vi "Station - Create New Station (SubVI).vi"(6 "Load?":bool, 8 "error constant":errorcluster, 10 "Test Type":u16(ring) items=["Please Select", "Triaxial Shear", "Triaxial UU", "Shearbox", "Permeability", "Consolidation (Stepped Loading)/Swelling", "Saturation (Incremental)", "User Defined", "UCT", "Isotropic Consolidation", "Swelling Pressure"], 11 "Station Name":string) -> (0 "error out":errorcluster, 2 "Station ID":string, 3 "ForceClose":bool=TRUE, 4 "Delete?":bool)   [LabVIEW 2019]
uses:
  Controls/Station name-state.ctl
  Controls/CreateStation - Data Structure.ctl
  Controls/Global - Device.vi
  Controls/Global - IP Address.vi
  Controls/Global - Data UDP.vi
  Controls/Global - Device Input.vi
  Controls/Global - Channel.vi
  Controls/Global - Unit.vi
panel:
  out "Device":string[](array[string])
  out "List":string[](array[string])
  in  "Cancel":bool
  in  "Delete":bool
  out "Sub Tab":T1(tab)
  in  "PP TS":u16(ring) caption="Vertical Load" items=["Please Select"]
  in  "Disp TS":u16(ring) caption="Back Pressure" items=["Please Select"]
  in  "LT TS":u16(ring) caption="Cell Pressure" items=["Please Select"]
  out "Unit PPT Triaxial Shear":string caption="Cell Pressure Transducer"
  out "Unit Disp Triaxial Shear":string caption="Cell Pressure Transducer"
  out "Unit LT Triaxial Shear":string caption="Cell Pressure Transducer"
  out "Unit VC Triaxial Shear":string caption="Cell Pressure Transducer"
  out "Unit BPT Triaxial Shear":string caption="Cell Pressure Transducer"
  out "Unit CPT Triaxial Shear":string caption="Cell Pressure Transducer"
  in  "VLC Triaxial Shear":u16(ring) caption="Vertical Load" items=["Please Select"]
  in  "BPC Triaxial Shear":u16(ring) caption="Back Pressure" items=["Please Select"]
  out "Disp Triaxial Shear":sgl caption="Displacement" format="%.3f"
  out "PPT Triaxial Shear":sgl caption="Pore Pressure"
  out "LT Triaxial Shear":sgl caption="Load"
  out "BPT Triaxial Shear":sgl caption="Back Pressure" format="%.3f"
  out "VC Triaxial Shear":sgl caption="Volume Change"
  out "CPT Triaxial Shear":sgl caption="Cell Pressure" format="%.3f"
  in  "VLC TS":u16(ring) caption="Vertical Load" items=["Please Select"]
  in  "BPC TS":u16(ring) caption="Back Pressure" items=["Please Select"]
  in  "CPC TS":u16(ring) caption="Cell Pressure" items=["Please Select"]
  in  "CPC Triaxial Shear":u16(ring) caption="Cell Pressure" items=["Please Select"]
  in  "PP TUU":u16(ring) caption="Vertical Load" items=["Please Select"]
  in  "Disp TUU":u16(ring) caption="Cell Pressure" items=["Please Select"]
  in  "VLC TUU":u16(ring) caption="Vertical Load" items=["Please Select"]
  in  "CPC TUU":u16(ring) caption="Cell Pressure" items=["Please Select"]
  out "Unit CPT Triaxial UU":string caption="Cell Pressure Transducer"
  out "Unit VLT Triaxial UU":string caption="Cell Pressure Transducer"
  out "Unit Disp Triaxial UU":string caption="Cell Pressure Transducer"
  out "Unit PPT Triaxial UU":string caption="Cell Pressure Transducer"
  in  "VLC Triaxial UU":u16(ring) caption="Vertical Load" items=["Please Select"]
  out "CPT Triaxial UU":sgl caption="Cell Pressure" format="%.5f"
  out "VLT Triaxial UU":sgl caption="Vertical Load" format="%.5f"
  out "PPT Triaxial UU":sgl caption="Pore Pressure" format="%.5f"
  out "Disp Triaxial UU":sgl caption="Displacement" format="%.5f"
  in  "CPC Triaxial UU":u16(ring) caption="Cell Pressure" items=["Please Select"]
  in  "HDisp Shearbox":u16(ring) caption="Horinzontal Load" items=["Please Select"]
  in  "HL Shearbox":u16(ring) caption="Vertical Load" items=["Please Select"]
  in  "VDisp Shearbox":u16(ring) caption="Horinzontal Load" items=["Please Select"]
  in  "VL Shearbox":u16(ring) caption="Vertical Load" items=["Please Select"]
  out "Unit LT Shearbox":string caption="Cell Pressure Transducer"
  out "Unit Disp Shearbox":string caption="Cell Pressure Transducer"
  out "Unit HLT Shearbox":string caption="Cell Pressure Transducer"
  out "Unit H Dis Shearbox":string caption="Cell Pressure Transducer"
  in  "HLC Shearbox":u16(ring) caption="Horinzontal Load" items=["Please Select"]
  out "LT Shearbox":sgl caption="V Load" format="%#.5f"
  out "Disp Shearbox":sgl caption="V Displacement" format="%#.5f"
  out "H Disp Shearbox":sgl caption="H Displacement" format="%#.5f"
  out "HLT Shearbox":sgl caption="H Load" format="%#.5f"
  in  "VLC Shearbox":u16(ring) caption="Vertical Load" items=["Please Select"]
  in  "OVC Permea":u16(ring) caption="Back Pressure 2" items=["Please Select"]
  in  "BP2 Permea":u16(ring) caption="Back Pressure" items=["Please Select"]
  in  "PP Permea":u16(ring) caption="Cell Pressure" items=["Please Select"]
  in  "IVC Permea":u16(ring) caption="Back Pressure 2" items=["Please Select"]
  in  "BP Permea":u16(ring) caption="Back Pressure" items=["Please Select"]
  in  "CP Permea":u16(ring) caption="Cell Pressure" items=["Please Select"]
  out "Unit CPT Permeability":string caption="Cell Pressure Transducer"
  out "Unit BPT Permeability":string caption="Cell Pressure Transducer"
  out "Unit IVC Permeability":string caption="Cell Pressure Transducer"
  out "Unit BPT2 Permeability":string caption="Cell Pressure Transducer"
  out "Unit OVC Permeability":string caption="Cell Pressure Transducer"
  out "Unit PPT Permeability":string caption="Cell Pressure Transducer"
  in  "BPC2 Permeability":u16(ring) caption="Drain Pressure" items=["Please Select"]
  in  "BPC Permeability":u16(ring) caption="Back Pressure" items=["Please Select"]
  out "BPT2 Permeability":sgl caption="Drain Pressure" format="%.5f"
  out "PPT Permeability":sgl caption="Pore Pressure" format="%.5f"
  out "OVC Permeability":sgl caption="Outlet VC" format="%.5f"
  out "BPT Permeability":sgl caption="Back Pressure" format="%.5f"
  out "IVC Permeability":sgl caption="Inlet VC" format="%.5f"
  out "CPT Permeability":sgl caption="Cell Pressure" format="%.5f"
  in  "CPC Permeability":u16(ring) caption="Cell Pressure" items=["Please Select"]
  in  "Disp Consol":u16(ring) caption="Vertical Load" items=["Please Select"]
  in  "LT Consol":u16(ring) caption="Vertical Load" items=["Please Select"]
  out "Unit LT Consolidation":string caption="Cell Pressure Transducer"
  out "Unit Disp Consolidation":string caption="Cell Pressure Transducer"
  out "Disp Consolidation":sgl caption="Displacement" format="%.5f"
  out "LT Consolidation":sgl caption="Load Tranducer" format="%.5f"
  in  "VLC Consolidation":u16(ring) caption="Vertical Load" items=["Please Select"]
  in  "VC Saturation":u16(ring) caption="Cell Pressure" items=["Please Select"]
  in  "PP Saturation":u16(ring) caption="Back Pressure" items=["Please Select"]
  in  "CP Saturation":u16(ring) caption="Cell Pressure" items=["Please Select"]
  in  "BP Saturation":u16(ring) caption="Back Pressure" items=["Please Select"]
  out "Unit CPT Saturation":string caption="Cell Pressure Transducer"
  out "Unit BPT Saturation":string caption="Cell Pressure Transducer"
  out "Unit VC Saturation":string caption="Cell Pressure Transducer"
  out "Unit PPT Saturation":string caption="Cell Pressure Transducer"
  out "CPT Saturation":sgl caption="Cell Pressure" format="%.1f"
  out "VC Saturation":sgl caption="Volume Change" format="%.1f"
  out "BPT Saturation":sgl caption="Back Pressure" format="%.1f"
  out "PPT Saturation":sgl caption="Pore pressure" format="%.1f"
  in  "CPC Saturation":u16(ring) caption="Cell Pressure" items=["Please Select"]
  in  "BPC Saturation":u16(ring) caption="Back Pressure" items=["Please Select"]
  in  "H Disp UD":u16(ring) caption="Horizontal Load" items=["Please Select"]
  in  "HL UD":u16(ring) caption="Vertical Load" items=["Please Select"]
  in  "VDisp UD":u16(ring) caption="Back Pressure 2" items=["Please Select"]
  in  "VL UD":u16(ring) caption="Back Pressure" items=["Please Select"]
  in  "VC2 UD":u16(ring) caption="Cell Pressure" items=["Please Select"]
  in  "BP2 UD":u16(ring) caption="Horizontal Load" items=["Please Select"]
  in  "PP UD":u16(ring) caption="Vertical Load" items=["Please Select"]
  in  "VC1 UD":u16(ring) caption="Back Pressure 2" items=["Please Select"]
  in  "BP UD":u16(ring) caption="Back Pressure" items=["Please Select"]
  in  "CP UD":u16(ring) caption="Cell Pressure" items=["Please Select"]
  out "HD User Defined":sgl caption="H Displacement" format="%.5f"
  out "HL User Defined":sgl caption="H Load" format="%.5f"
  out "VD User Defined":sgl caption="V Displacement" format="%.5f"
  out "VC2 User Defined":sgl caption="Volume Change 2" format="%.5f"
  out "VC1 User Defined":sgl caption="Volume Change 1" format="%.5f"
  out "VL User Defined":sgl caption="V Load" format="%.5f"
  out "BPT2 User Defined":sgl caption="Drain Pressure" format="%.5f"
  out "PWP User Defined":sgl caption="Pore Pressure" format="%.5f"
  out "BPT User Defined":sgl caption="Back Pressure" format="%.5f"
  out "CPT User Defined":sgl caption="Cell Pressure" format="%.5f"
  in  "HLC User Defined":u16(ring) caption="Horizontal Load" items=["Please Select"]
  in  "VLC User Defined":u16(ring) caption="Vertical Load" items=["Please Select"]
  in  "BPC2 User Defined":u16(ring) caption="Drain Pressure" items=["Please Select"]
  in  "BPC User Defined":u16(ring) caption="Back Pressure" items=["Please Select"]
  in  "CPC User Defined":u16(ring) caption="Cell Pressure" items=["Please Select"]
  out "Unit VL User Defined":string caption="Cell Pressure Transducer"
  out "Unit VD User Defined":string caption="Cell Pressure Transducer"
  out "Unit HL User Defined":string caption="Cell Pressure Transducer"
  out "Unit HD User Defined":string caption="Cell Pressure Transducer"
  out "Unit VC2 User Defined":string caption="Cell Pressure Transducer"
  out "Unit BPT2 User Defined":string caption="Cell Pressure Transducer"
  out "Unit PWP User Defined":string caption="Cell Pressure Transducer"
  out "Unit VC1 User Defined":string caption="Cell Pressure Transducer"
  out "Unit BPT User Defined":string caption="Cell Pressure Transducer"
  out "Unit CPT User Defined":string caption="Cell Pressure Transducer"
  in  "Disp UCT":u16(ring) caption="Vertical Load" items=["Please Select"]
  in  "LT UCT":u16(ring) caption="Vertical Load" items=["Please Select"]
  out "Unit LT UCT":string caption="Cell Pressure Transducer"
  out "Unit Disp UCT":string caption="Cell Pressure Transducer"
  out "Disp iUCT":sgl caption="Displacement"
  out "LT iUCT":sgl caption="Load Tranducer"
  in  "VLC UCT":u16(ring) caption="Vertical Load" items=["Please Select"]
  in  "VC IsoCons":u16(ring) caption="Cell Pressure" items=["Please Select"]
  in  "PP IsoCons":u16(ring) caption="Back Pressure" items=["Please Select"]
  in  "CP IsoCons":u16(ring) caption="Cell Pressure" items=["Please Select"]
  in  "BP IsoCons":u16(ring) caption="Back Pressure" items=["Please Select"]
  out "Unit CPT IsoCons":string caption="Cell Pressure Transducer"
  out "Unit BPT IsoCons":string caption="Cell Pressure Transducer"
  out "Unit VC IsoCons":string caption="Cell Pressure Transducer"
  out "Unit PPT IsoCons":string caption="Cell Pressure Transducer"
  out "CPT iIsoCons":sgl caption="Cell Pressure" format="%.1f"
  out "VC iIsoCons":sgl caption="Volume Change"
  out "BPT iIsoCons":sgl caption="Back Pressure"
  out "PPT iIsoCons":sgl caption="Pore pressure"
  in  "CPC IsoCons":u16(ring) caption="Cell Pressure" items=["Please Select"]
  in  "BPC IsoCons":u16(ring) caption="Back Pressure" items=["Please Select"]
  in  "VL SPres":u16(ring) caption="Cell Pressure" items=["Please Select"]
  in  "VS SPress":u16(ring) caption="Back Pressure" items=["Please Select"]
  out "Unit VL SP":string caption="Cell Pressure Transducer"
  out "Unit VS SP":string caption="Cell Pressure Transducer"
  out "VL SP":sgl caption="Vertical Load" format="%.1f"
  out "VS SP":sgl caption="Vertical Stress"
  in  "Save":bool
  # "Live Reading"
  # "Control"
  # "Display"
  # "Live Reading"
  # "Display"
  # "Control"
  # "Live Reading"
  # "Control"
  # "Display"
  # "Live Reading"
  # "Control"
  # "Display"
  # "Live Reading"
  # "Control"
  # "Display"
  # "Live Reading"
  # "Control"
  # "Display"
  # "Display"
  # "Control"
  # "Live Reading"
  # "Control"
  # "Display"
  # "Live Reading"
  # "Control"
  # "Display"
  # "Live Reading"
  # "Control"
  # "Display"
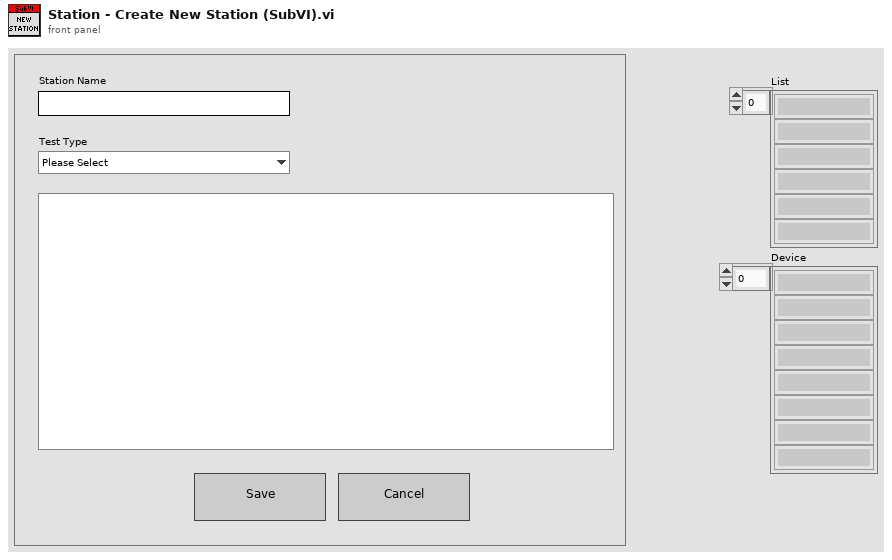
[diagram p1: front panel]
types:
  T1 = enum32{"Please Select", "Triaxial Shear", "Triaxial UU", "Shearbox", "Permeability", "Consolidation", "Saturation", "User Defined", "UCT", "Iso Consolidation", "Swelling Pressure"}
  T2 = enum16{"open", "replace", "create", "open or create", "replace or create", "replace or create with confirmation"}
  T3 = typedef "Station name-state.ctl" = enum16{"Init", "Idle", "Save", "Load", "Read", "Close"}
  T4 = typedef "CreateStation - Data Structure.ctl" = cluster{"Station Name":string[], "Station ID":i32}
  T5 = enum8{"Enabled", "Disabled", "Disabled and Grayed Out"}
  T6 = enum32{"Please Select", "Triaxial Shear", "Triaxial UU", "Shearbox", "Permeability", "Consolidation", "Saturation", "User Defined"}
  T7 = cluster{"Station Name":string, "Key Value":string[], "Key Names":string[]}[]
  T8 = typedef "UDP - Event.ctl" = u16
  T9 = typedef "UDP - Status.ctl" = u16
  T10 = cluster{"Channels":cluster{"Ch1":sgl, "Ch2":sgl, "Ch3":sgl, "Ch4":sgl, "Ch5":sgl, "Ch6":sgl, "Ch7":sgl, "Ch8":sgl, "Ch9":sgl, "Ch10":sgl, "Ch11":sgl, "Ch12":sgl, "Ch13":sgl, "Ch14":sgl, "Ch15":sgl, "Ch16":sgl}, "Event":T8, "Status":T9, "IP":string}[]
  T11 = cluster{"Name":string[], "Unit":string[], "Decimal Point":u8[], "Ch Log":u8[], "H Alarm":u8[], "L Alarm":u8[], "H Limit":sgl[], "L Limit":sgl[], "Filter":u8[], "Gain":u8[], "Calib Type":u32[]}[]
  T12 = cluster{"Channels":cluster{"Ch1":sgl, "Ch2":sgl, "Ch3":sgl, "Ch4":sgl, "Ch5":sgl, "Ch6":sgl, "Ch7":sgl, "Ch8":sgl, "Ch9":sgl, "Ch10":sgl, "Ch11":sgl, "Ch12":sgl, "Ch13":sgl, "Ch14":sgl, "Ch15":sgl, "Ch16":sgl}, "Event":T8, "Status":T9, "IP":string}
  T13 = cluster{"Name":string[], "Unit":string[], "Decimal Point":u8[], "Ch Log":u8[], "H Alarm":u8[], "L Alarm":u8[], "H Limit":sgl[], "L Limit":sgl[], "Filter":u8[], "Gain":u8[], "Calib Type":u32[]}
  T14 = cluster{"Ch1":sgl, "Ch2":sgl, "Ch3":sgl, "Ch4":sgl, "Ch5":sgl, "Ch6":sgl, "Ch7":sgl, "Ch8":sgl, "Ch9":sgl, "Ch10":sgl, "Ch11":sgl, "Ch12":sgl, "Ch13":sgl, "Ch14":sgl, "Ch15":sgl, "Ch16":sgl}
  T15 = cluster{"Station Name":string, "Key Value":string[], "Key Names":string[]}
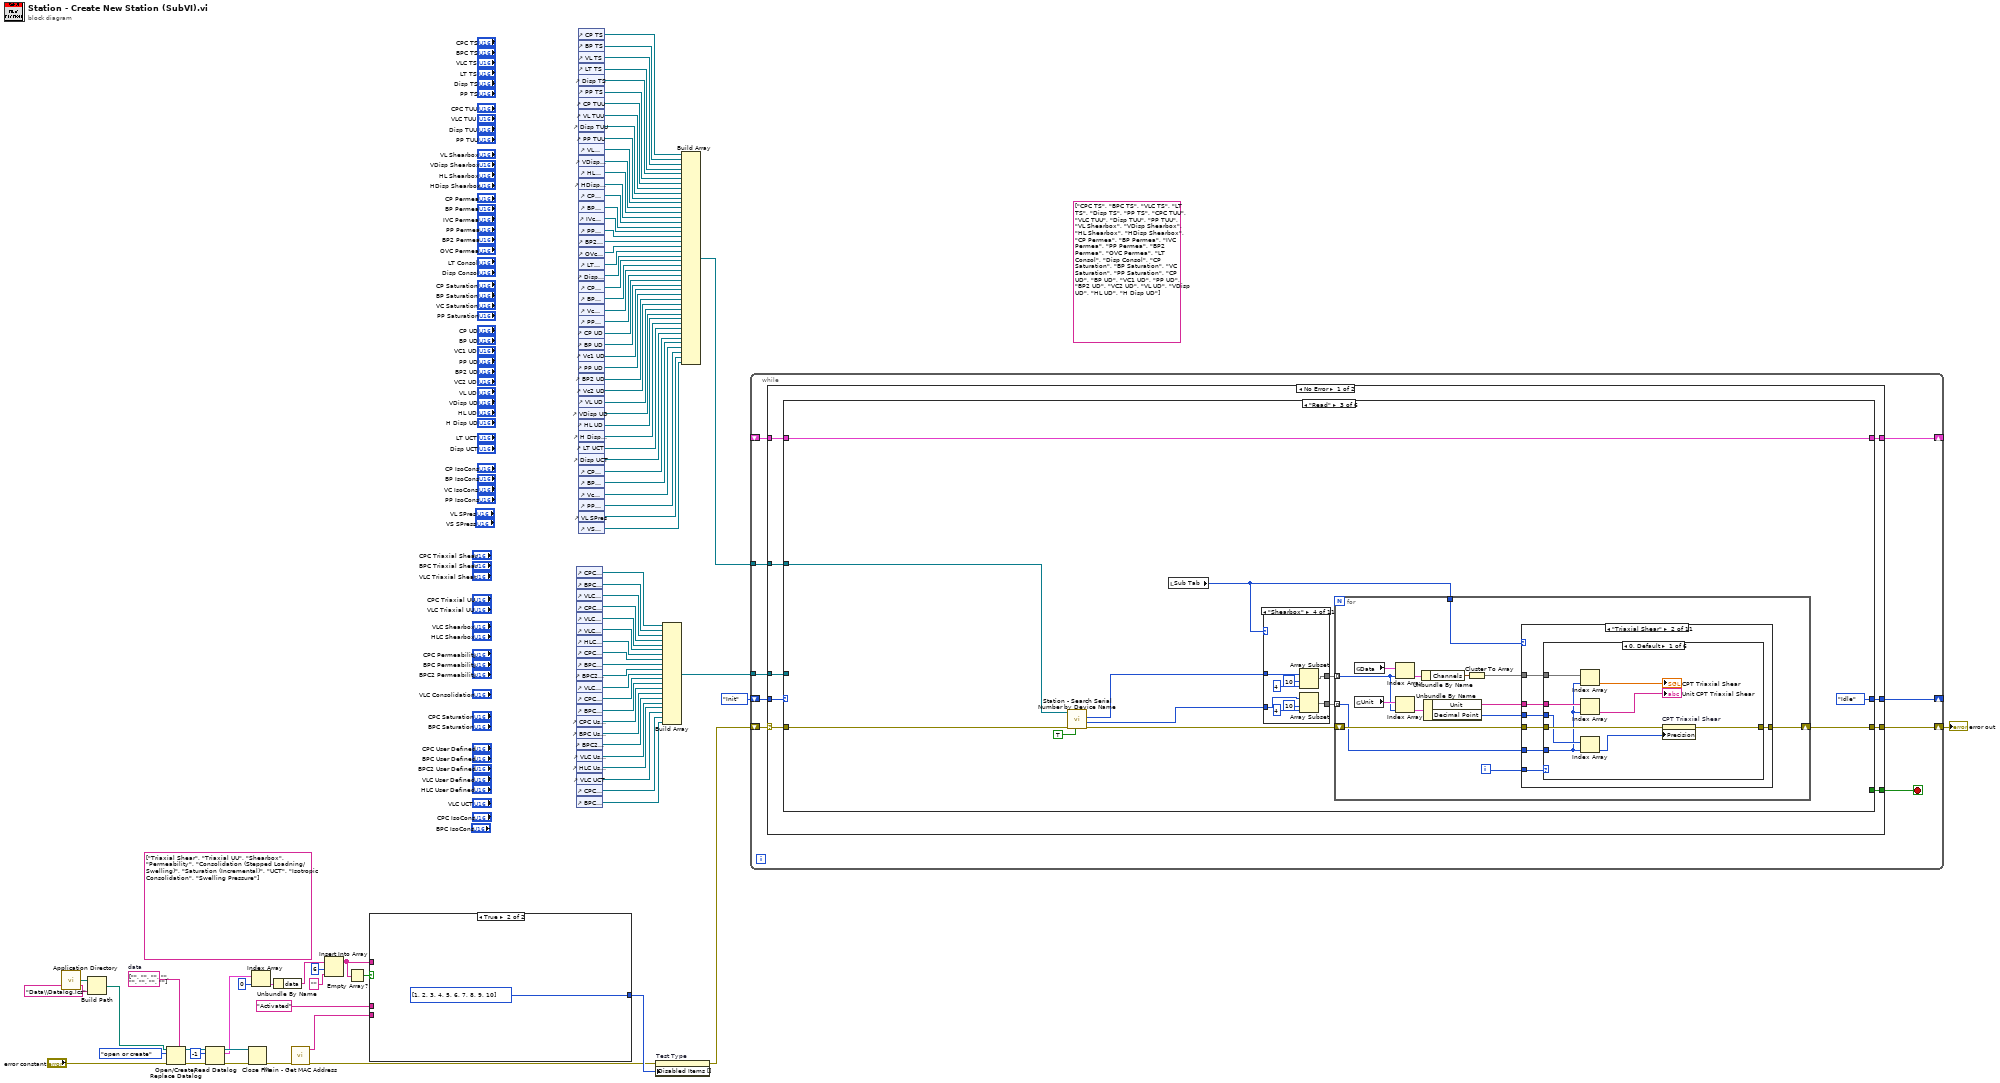
[diagram p0: block diagram]
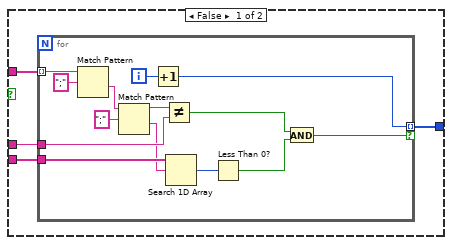
[diagram p2: hidden frame]
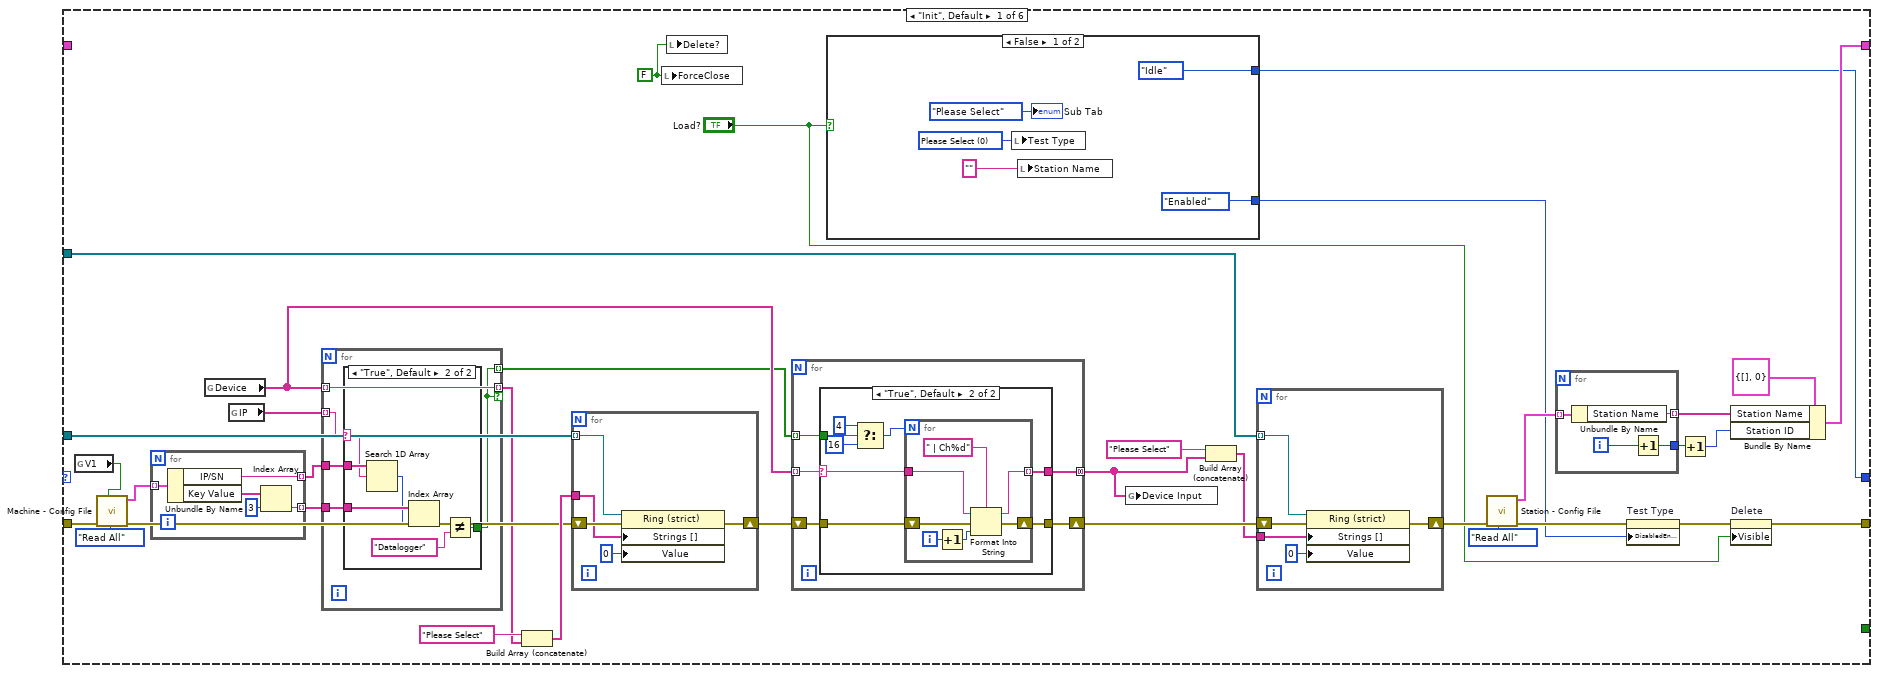
[diagram p3: hidden frame]
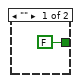
[diagram p4: hidden frame]
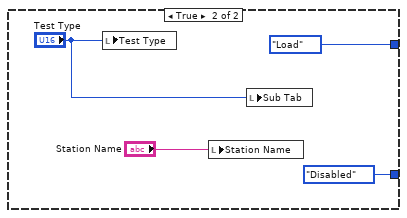
[diagram p5: hidden frame]
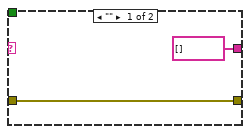
[diagram p6: hidden frame]
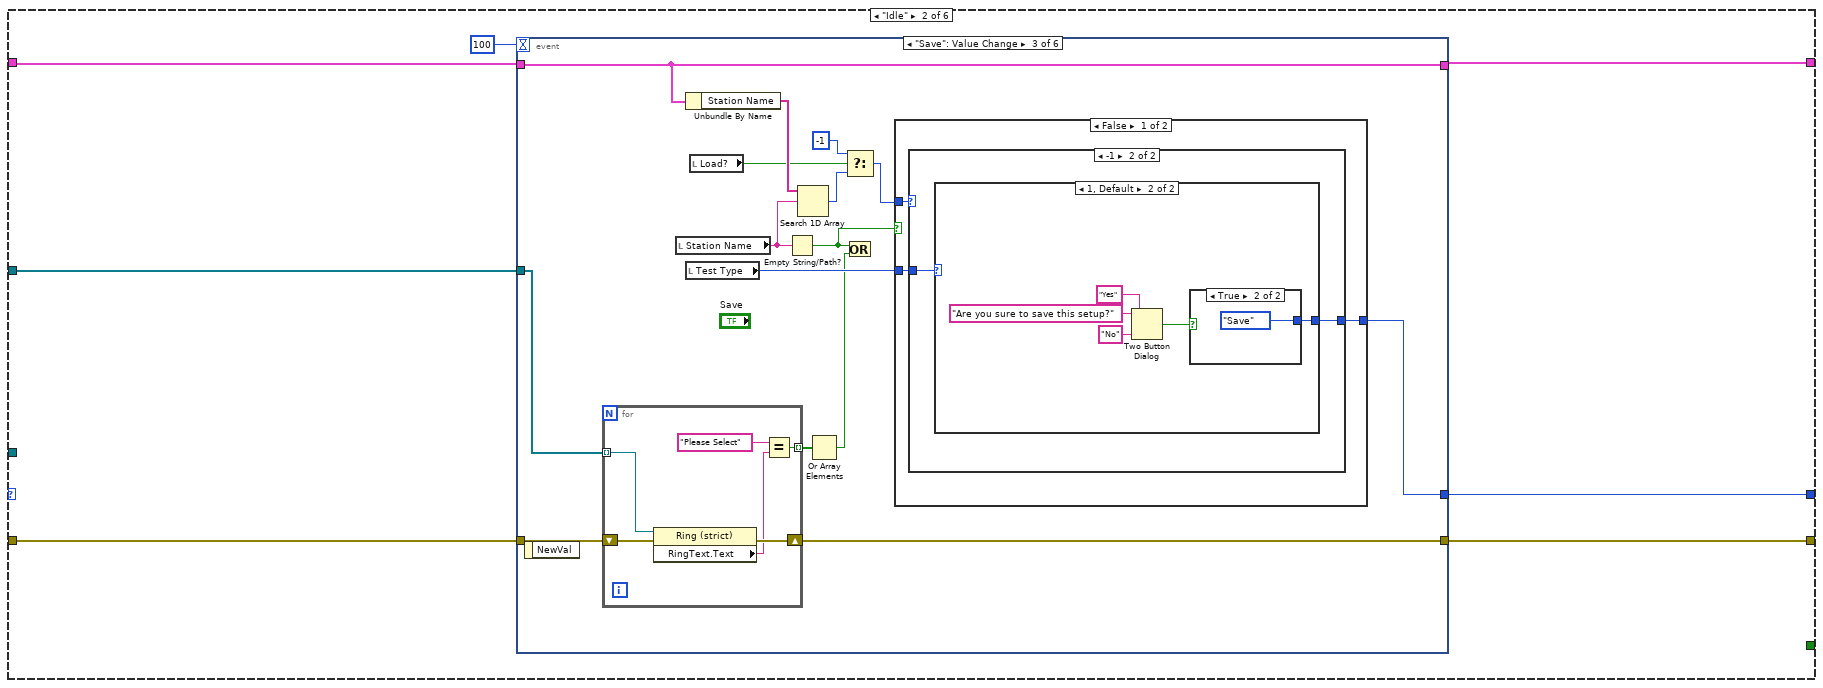
[diagram p7: hidden frame]
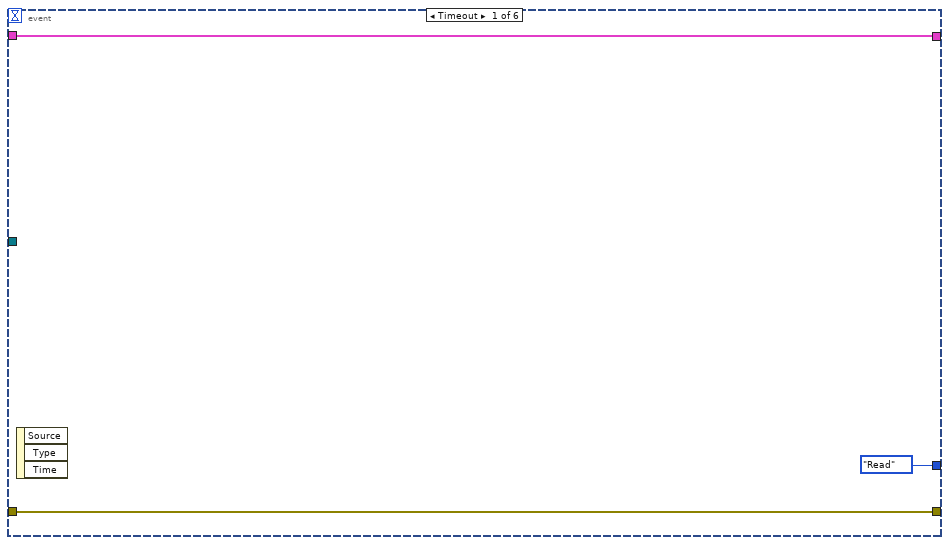
[diagram p8: hidden frame]
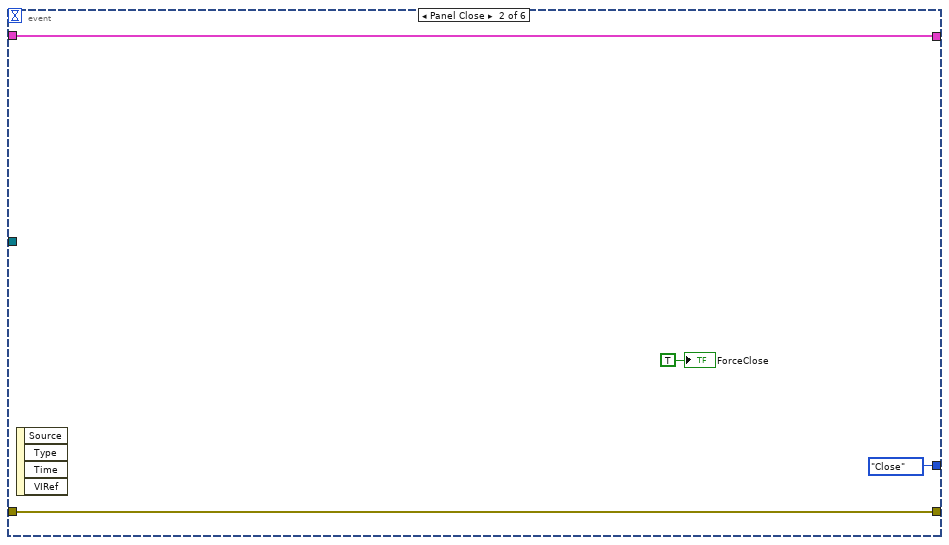
[diagram p9: hidden frame]
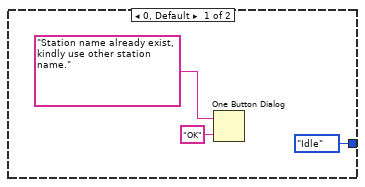
[diagram p10: hidden frame]
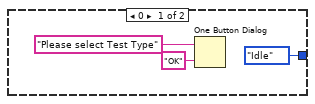
[diagram p11: hidden frame]
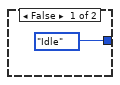
[diagram p12: hidden frame]
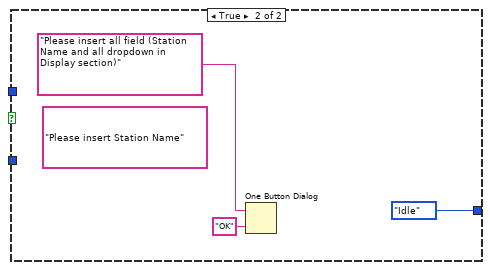
[diagram p13: hidden frame]
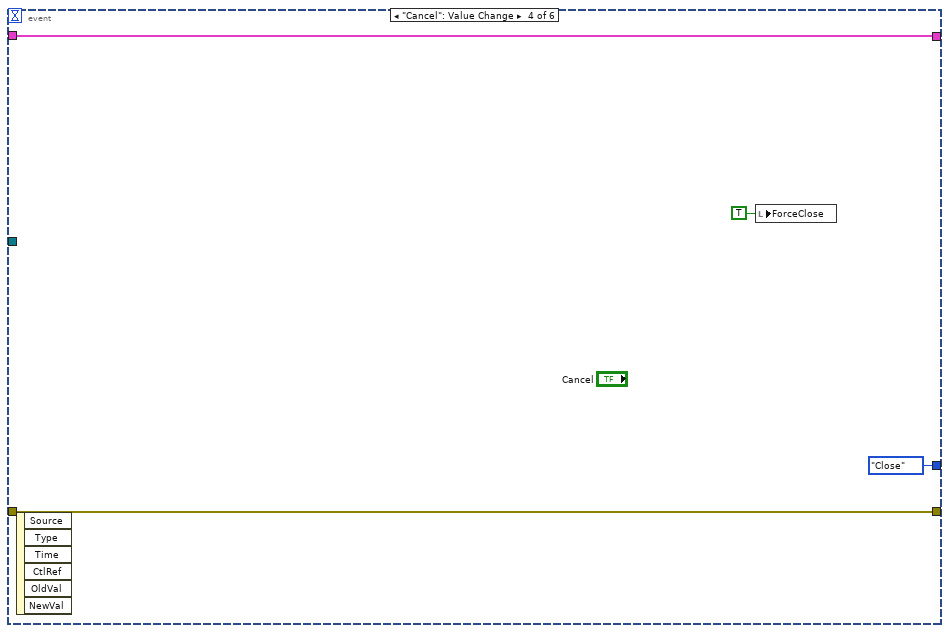
[diagram p14: hidden frame]
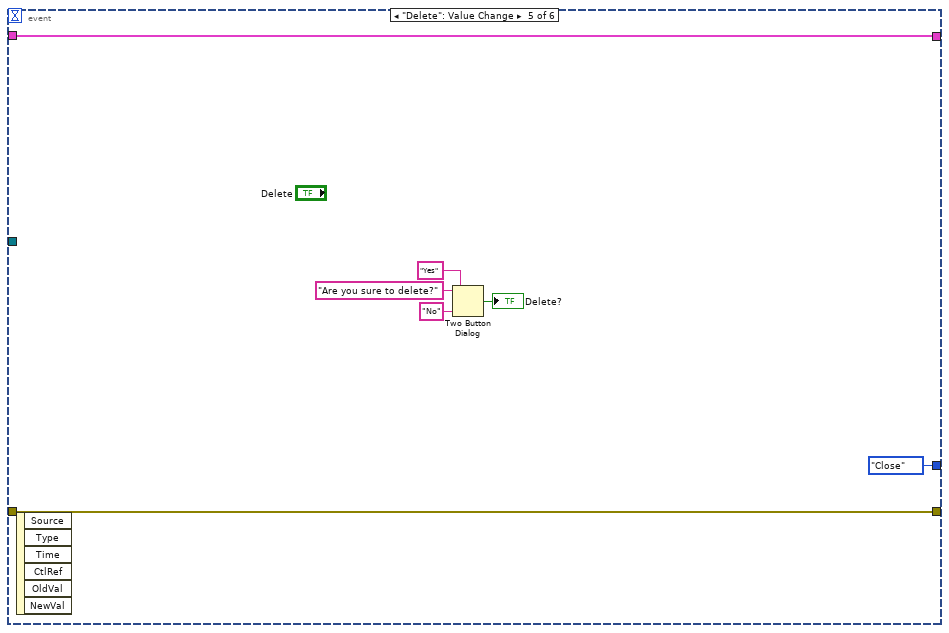
[diagram p15: hidden frame]
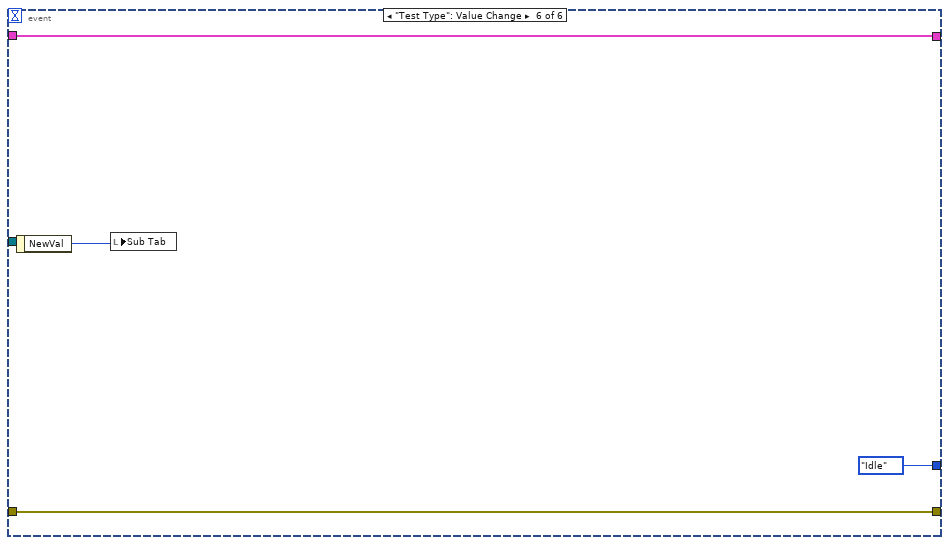
[diagram p16: hidden frame]
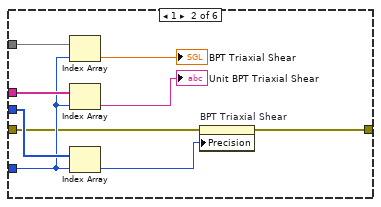
[diagram p18: hidden frame]
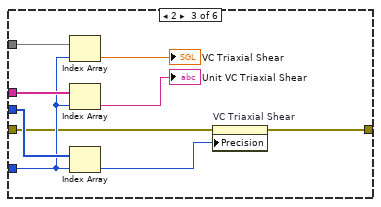
[diagram p19: hidden frame]
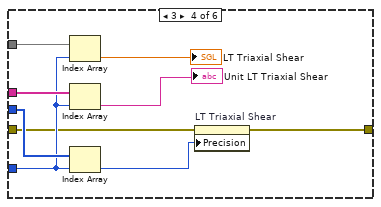
[diagram p20: hidden frame]
diagram:
  (unwired) string[] ["Triaxial Shear", "Triaxial UU", "Shearbox", "Permeability", "Consolidation (Stepped Loadning/Swelling)", "Saturation (Incremental)", "UCT", "Isotropic Consolidation", "Swelling Pressure"]
  w23 = string[] ["", "", "", "", "", "", "", ""]  # data
  (unwired) string[] ["CPC TS", "BPC TS", "VLC TS", "LT TS", "Disp TS", "PP TS", "CPC TUU", "VLC TUU", "Disp TUU", "PP TUU", "VL Shearbox", "VDisp Shearbox", "HL Shearbox", "HDisp Shearbox", "CP Permea", "BP Permea", "IVC Permea", "PP Permea", "BP2 Permea", "OVC Permea", "LT Consol", "Disp Consol", "CP Saturation", "BP Saturation", "VC Saturation", "PP Saturation", "CP UD", "BP UD", "VC1 UD", "PP UD", "BP2 UD", "VC2 UD", "VL UD", "VDisp UD", "HL UD", "H Disp UD"] ("Array")
  n1 = call <vilib>:"Application Directory.vi"() -> ("Application Directory"=w27:path)
  n2 = Build Path(base path=w27, name or relative path="Data\\Datalog.lcs") -> (appended path=w15:path)
  n3 = Open/Create/Replace Datalog(5:w23, 8:"error constant", 10:T2."open or create" ("operation (0:open)"), 11:w15) -> (0:w25:errorcluster, 3:w22:refnum<k1>)  [unwired: 2 in, 1 out]
  n4 = Read Datalog(4:w25, 6:-1 ("count (1)"), 7:w22) -> (0:w24:errorcluster, 2:w18:cluster{"data":string[]}[], 3:w21:refnum<k1>)
  n5 = Close File(refnum=w21, error in=w24) -> (error out=w5:errorcluster)  [unwired: 1 out]
  n6 = Index Array(array=w18, index=0) -> (element=w16:cluster{"data":string[]})
  n7 = Unbundle By Name(w16) -> ("data"=w10:string[])
  n8 = call "Main - Get MAC Address.vi"("error in (no error)"=w5) -> ("error out"=w4:errorcluster, "MAC Address"=w3:string[])  [unwired: 9 in]
  n9 = Insert Into Array(array=w10, index=6, new element="" ("new element/subarray")) -> (w7:string[])
  n10 = Empty Array?(array=w7) -> (empty?=w6:bool)
  n11 = case shown="True" w6 {
    tunnel: "Activated" -> [w98 _]
    tunnel: [w97 i32[] [1, 2, 3, 4, 5, 6, 7, 8, 9, 10]] -> w11
    tunnel: w7 -> [w96 _]
    tunnel: w3 -> [w95 _]
    frame False {
      n12 = for {
        tunnel: w96 -> [w108] mode=indexing
        tunnel: w98 -> [w112]
        tunnel: [w110] -> w97 mode=indexing if=w99
        tunnel: w95 -> [w104]
        i -> [w111]
        n13 = Match Pattern(string=w108, regular expression=";") -> (after substring=w106:string)  [unwired: 1 in, 3 out]
        n14 = Match Pattern(string=w106, regular expression=";") -> (before substring=w105:string, after substring=w103:string)  [unwired: 1 in, 2 out]
        n15 = Increment(x=w111) -> (x+1=w110:i32)
        n16 = Not Equal?(x=w105, y=w112) -> (x != y?=w100:bool)
        n17 = Search 1D Array(1D array=w104, element=w103) -> (index of element=w102:i32)  [unwired: 1 in]
        n18 = Less Than 0?(x=w102) -> (x < 0?=w101:bool)
        n19 = And(x=w100, y=w101) -> (x .and. y?=w99:bool)
      }
    }
    frame True {
    }
  }
  n20 = control-ref of="CPC Triaxial Shear"() -> (w93:refnum<vi>)
  n21 = control-ref of="BPC Triaxial Shear"() -> (w92:refnum<vi>)
  n22 = control-ref of="VLC Triaxial Shear"() -> (w91:refnum<vi>)
  n23 = control-ref of="CPC Triaxial UU"() -> (w90:refnum<vi>)
  n24 = control-ref of="VLC Triaxial UU"() -> (w89:refnum<vi>)
  n25 = control-ref of="VLC Shearbox"() -> (w88:refnum<vi>)
  n26 = control-ref of="HLC Shearbox"() -> (w87:refnum<vi>)
  n27 = control-ref of="CPC Permeability"() -> (w86:refnum<vi>)
  n28 = control-ref of="BPC Permeability"() -> (w85:refnum<vi>)
  n29 = control-ref of="BPC2 Permeability"() -> (w84:refnum<vi>)
  n30 = control-ref of="VLC Consolidation"() -> (w83:refnum<vi>)
  n31 = control-ref of="CPC Saturation"() -> (w82:refnum<vi>)
  n32 = control-ref of="BPC Saturation"() -> (w81:refnum<vi>)
  n33 = control-ref of="CPC User Defined"() -> (w80:refnum<vi>)
  n34 = control-ref of="BPC User Defined"() -> (w79:refnum<vi>)
  n35 = control-ref of="BPC2 User Defined"() -> (w78:refnum<vi>)
  n36 = control-ref of="VLC User Defined"() -> (w77:refnum<vi>)
  n37 = control-ref of="HLC User Defined"() -> (w76:refnum<vi>)
  n38 = control-ref of="VLC UCT"() -> (w36:refnum<vi>)
  n39 = control-ref of="CPC IsoCons"() -> (w35:refnum<vi>)
  n40 = control-ref of="BPC IsoCons"() -> (w34:refnum<vi>)
  n41 = control-ref of="CP TS"() -> (w75:refnum<vi>)
  n42 = control-ref of="BP TS"() -> (w74:refnum<vi>)
  n43 = control-ref of="VL TS"() -> (w73:refnum<vi>)
  n44 = control-ref of="LT TS"() -> (w72:refnum<vi>)
  n45 = control-ref of="Disp TS"() -> (w71:refnum<vi>)
  n46 = control-ref of="PP TS"() -> (w70:refnum<vi>)
  n47 = control-ref of="CP TUU"() -> (w69:refnum<vi>)
  n48 = control-ref of="VL TUU"() -> (w68:refnum<vi>)
  n49 = control-ref of="Disp TUU"() -> (w67:refnum<vi>)
  n50 = control-ref of="PP TUU"() -> (w66:refnum<vi>)
  n51 = control-ref of="VL Shearbox"() -> (w65:refnum<vi>)
  n52 = control-ref of="VDisp Shearbox"() -> (w64:refnum<vi>)
  n53 = control-ref of="HL Shearbox"() -> (w63:refnum<vi>)
  n54 = control-ref of="HDisp Shearbox"() -> (w62:refnum<vi>)
  n55 = control-ref of="CP Permea"() -> (w61:refnum<vi>)
  n56 = control-ref of="BP Permea"() -> (w60:refnum<vi>)
  n57 = control-ref of="IVc Permea"() -> (w59:refnum<vi>)
  n58 = control-ref of="PP Permea"() -> (w58:refnum<vi>)
  n59 = control-ref of="BP2 Permea"() -> (w57:refnum<vi>)
  n60 = control-ref of="OVc Permea"() -> (w56:refnum<vi>)
  n61 = control-ref of="LT Consol"() -> (w55:refnum<vi>)
  n62 = control-ref of="Disp Consol"() -> (w54:refnum<vi>)
  n63 = control-ref of="CP Saturation"() -> (w53:refnum<vi>)
  n64 = control-ref of="BP Saturation"() -> (w52:refnum<vi>)
  n65 = control-ref of="Vc Saturation"() -> (w51:refnum<vi>)
  n66 = control-ref of="PP Saturation"() -> (w50:refnum<vi>)
  n67 = control-ref of="CP UD"() -> (w49:refnum<vi>)
  n68 = control-ref of="BP UD"() -> (w48:refnum<vi>)
  n69 = control-ref of="Vc1 UD"() -> (w47:refnum<vi>)
  n70 = control-ref of="PP UD"() -> (w46:refnum<vi>)
  n71 = control-ref of="BP2 UD"() -> (w45:refnum<vi>)
  n72 = control-ref of="Vc2 UD"() -> (w44:refnum<vi>)
  n73 = control-ref of="VL UD"() -> (w43:refnum<vi>)
  n74 = control-ref of="VDisp UD"() -> (w42:refnum<vi>)
  n75 = control-ref of="HL UD"() -> (w41:refnum<vi>)
  n76 = control-ref of="H Disp UD"() -> (w40:refnum<vi>)
  n77 = control-ref of="LT UCT"() -> (w33:refnum<vi>)
  n78 = control-ref of="Disp UCT"() -> (w32:refnum<vi>)
  n79 = control-ref of="CP IsoCons"() -> (w31:refnum<vi>)
  n80 = control-ref of="BP IsoCons"() -> (w30:refnum<vi>)
  n81 = control-ref of="Vc IsoCons"() -> (w29:refnum<vi>)
  n82 = control-ref of="PP IsoCons"() -> (w28:refnum<vi>)
  n83 = control-ref of="VL SPres"() -> (w2:refnum<vi>)
  n84 = control-ref of="VS SPress"() -> (w1:refnum<vi>)
  n85 = property on="Test Type" class="Ring (strict)"(error in=w4, "Disabled Items []"=w11) -> (error out=w13:errorcluster)  [unwired: 1 in, 1 out]
  n86 = Build Array(w93, w92, w91, w90, w89, w88, w87, w86, w85, w84, w83, w82, w81, w80, w79, w78, w77, w76, w36, w35, w34) -> (w94:refnum<vi>[])
  n87 = Build Array(w75, w74, w73, w72, w71, w70, w69, w68, w67, w66, w65, w64, w63, w62, w61, w60, w59, w58, w57, w56, w55, w54, w53, w52, w51, w50, w49, w48, w47, w46, w45, w44, w43, w42, w41, w40, w33, w32, w31, w30, w29, w28, w2, w1) -> (w39:refnum<vi>[])
  n88 = while {
    shift-right: [w121] -> w37
    shift-left: w13 -> [w122]
    shift-right: [w119] -> _
    shift-left: Station_name-state."Init" -> [w120]
    shift-right: [w118] -> _
    shift-left: _ -> [w117]
    tunnel: w94 -> [w115]
    tunnel: w39 -> [w114]
    stop <- w116 stop-if-true
    n89 = case shown="No Error" w122 {
      selector: w122 -> [w131 w1207]
      tunnel: [w130 w1207] -> w121
      tunnel: w120 -> [w129 _]
      tunnel: [w128 _] -> w119
      tunnel: [w127 _] -> w118
      tunnel: w117 -> [w126 _]
      tunnel: [w125 _] -> w116
      tunnel: w115 -> [w124 _]
      tunnel: w114 -> [w123 _]
      frame No Error {
        n90 = case shown="\"Read\"" w129 {
          tunnel: w131 -> [w139 w236 w310 w896 w1055 w1206]
          tunnel: [w146 w235 w307 w902 w1052 w1206] -> w130
          tunnel: [w150 w234 Station_name-state."Idle" w901 Station_name-state."Idle" Station_name-state."Close"] -> w128
          tunnel: [w162 w232 w312 w886 w1053 T4 {"Station Name"=[], "Station ID"=0}] -> w127
          tunnel: w126 -> [_ w233 w312 w886 w1053 _]
          tunnel: [_ _ _ _ _ TRUE] -> w125
          tunnel: w124 -> [w166 _ _ w895 w1050 _]
          tunnel: w123 -> [w155 w230 w304 w877 w1049 _]
          frame "Init", Default {
            w144 = FALSE ("ForceClose")
            n91 = global read "Global - Data UDP.vi" "V1"() -> (w132:bool)
            n92 = call "Machine - Config File.vi"("Action"=enum16{"Write", "Read", "Read All", "Remove"}."Read All", "V1"=w132, "error in (no error)"=w139) -> ("error out"=w140:errorcluster, "Value Out"=w142:cluster{"IP/SN":string, "Key Value":string[]}[])  [unwired: 7 in]
            n93 = for {
              tunnel: w142 -> [w182] mode=indexing
              tunnel: [w181] -> w136 mode=indexing
              tunnel: [w180] -> w137 mode=indexing
              n94 = Unbundle By Name(w182) -> ("IP/SN"=w180:string, "Key Value"=w184:string[])
              n95 = Index Array(array=w184, index=3) -> (element=w181:string)
            }
            n96 = global read "Global - Device.vi" "Device"() -> (w134:string[])
            n97 = global read "Global - IP Address.vi" "IP"() -> (w138:string[])
            n98 = for {
              tunnel: w138 -> [w167] mode=indexing
              tunnel: w134 -> [w169] mode=indexing
              tunnel: w137 -> [w171]
              tunnel: w136 -> [w170]
              tunnel: [w169] -> w135 mode=indexing if=w168
              tunnel: [w168] -> w133 mode=indexing
              n99 = case shown="\"True\", Default" w167 {
                selector: w167 -> [_ w173]
                tunnel: w171 -> [_ w179]
                tunnel: w170 -> [_ w178]
                tunnel: [FALSE w174] -> w168
                frame "" {
                }
                frame "True", Default {
                  n100 = Search 1D Array(1D array=w179, element=w173) -> (index of element=w177:i32)  [unwired: 1 in]
                  n101 = Index Array(array=w178, index=w177) -> (element=w176:string)
                  n102 = Not Equal?(x=w176, y="Datalogger") -> (x != y?=w174:bool)
                }
              }
            }
            n103 = Build Array (concatenate)("Please Select", w135) -> (w159:string[])
            n104 = for {
              shift-right: [w228] -> w153
              shift-left: w140 -> [w229]
              tunnel: w166 -> [w227] mode=indexing
              tunnel: w159 -> [w225]
              n105 = property class="Ring (strict)"(reference=w227, error in=w229, "Strings []"=w225, "Value"=u16 0) -> (error out=w228:errorcluster)  [unwired: 1 out]
            }
            n106 = local write "ForceClose"(w144) -> ()
            n107 = local write "Delete?"(w144) -> ()
            n108 = for {
              tunnel: w134 -> [w194] mode=indexing
              shift-right: [w196] -> w152
              shift-left: w153 -> [w198]
              tunnel: [w197] -> w143 mode=concatenating
              tunnel: w133 -> [w195] mode=indexing
              n109 = case shown="\"True\", Default" w194 {
                selector: w194 -> [_ w201]
                tunnel: w198 -> [w200 w208]
                tunnel: [string[] [] w207] -> w197
                tunnel: [w200 w206] -> w196
                tunnel: w195 -> [_ w205]
                frame "" {
                }
                frame "True", Default {
                  n110 = Select(t=4, s=w205, f=16) -> (s? t:f=w202:i32)
                  n111 = for {
                    N: w202 -> [_]
                    shift-right: [w212] -> w206
                    shift-left: w208 -> [w213]
                    tunnel: w201 -> [w210]
                    tunnel: [w209] -> w207 mode=indexing
                    i -> [w211]
                    n112 = Increment(x=w211) -> (x+1=w215:i32)
                    n113 = Format Into String(format string=" | Ch%d", initial string=w210, error in=w213, w215) -> (resulting string=w209:string, error out=w212:errorcluster)
                  }
                }
              }
            }
            n114 = case shown="False" "Load?" {
              tunnel: [Station_name-state."Idle" Station_name-state."Load"] -> w150
              tunnel: [T5."Enabled" ("Disabled") T5."Disabled" ("Disabled")] -> w148
              frame False {
                w185 = u16 0 items=["Please Select", "Triaxial Shear", "Triaxial UU", "Shearbox", "Permeability", "Consolidation (Stepped Loading)/Swelling", "Saturation (Incremental)", "User Defined", "UCT", "Isotropic Consolidation"] ("Test Type")
                n115 = local write "Test Type"(w185) -> ()
                n116 = local write "Station Name"("" ("Give a Name for the Station")) -> ()
                "Sub Tab" <- T6."Please Select" ("Sub Tab")
              }
              frame True {
                n117 = local write "Test Type"("Test Type") -> ()
                n118 = local write "Station Name"("Station Name") -> ()
                n119 = local write "Sub Tab"("Test Type") -> ()
              }
            }
            n120 = global write "Global - Device Input.vi" "Device Input"(w143) -> ()
            n121 = Build Array (concatenate)("Please Select", w143) -> (w151:string[])
            n122 = for {
              shift-right: [w219] -> w156
              shift-left: w152 -> [w220]
              tunnel: w155 -> [w218] mode=indexing
              tunnel: w151 -> [w216]
              n123 = property class="Ring (strict)"(reference=w218, error in=w220, "Strings []"=w216, "Value"=u16 0) -> (error out=w219:errorcluster)  [unwired: 1 out]
            }
            n124 = call "Station - Config File.vi"("Action"=enum16{"Write", "Read", "Read All", "Remove"}."Read All", "error in (no error)"=w156) -> ("error out"=w149:errorcluster, "Value Out"=w164:T7)  [unwired: 8 in]
            n125 = for {
              tunnel: w164 -> [w224] mode=indexing
              tunnel: [w223] -> w161 mode=indexing
              tunnel: [w221] -> w158
              i -> [w222]
              n126 = Unbundle By Name(w224) -> ("Station Name"=w223:string)
              n127 = Increment(x=w222) -> (x+1=w221:i32)
            }
            n128 = property on="Test Type" class="Ring (strict)"(error in=w149, "DisabledEnum"=w148) -> (error out=w147:errorcluster)  [unwired: 1 in, 1 out]
            n129 = Increment(x=w158) -> (x+1=w157:i32)
            n130 = Bundle By Name(cluster=T4 {"Station Name"=[], "Station ID"=0}, "Station Name"=w161, "Station ID"=w157) -> (w162:T4)
            n131 = property on="Delete" class="Bool"(error in=w147, "Visible"="Load?") -> (error out=w146:errorcluster)  [unwired: 1 in, 1 out]
          }
          frame "Idle" {
            n132 = event shown="[2] \"Save\": Value Change" {
              selector: _ -> [_ _ _ _ _ _]
              dyn-events: _ -> [_ _ _ _ _ _]
              timeout: 100 -> [_ _ _ _ _ _]
              tunnel: w236 -> [w239 w243 w248 w289 w296 w298]
              tunnel: [w239 w243 w249 w289 w296 w298] -> w235
              tunnel: [Station_name-state."Read" Station_name-state."Close" w258 Station_name-state."Close" Station_name-state."Close" Station_name-state."Idle"] -> w234
              tunnel: w233 -> [w237 w242 w255 w288 w295 w299]
              tunnel: [w237 w242 w255 w288 w295 w299] -> w232
              tunnel: w230 -> [_ _ w247 _ _ _]
              event Timeout {
                n133 = event-data() -> ()  [unwired: 1 in, 3 out]
              }
              event Panel Close {
                n134 = event-data() -> ()  [unwired: 1 in, 4 out]
                "ForceClose" <- TRUE
              }
              event "Save": Value Change {
                n135 = event-data() -> ()  [unwired: 1 in, 1 out]
                n136 = for {
                  shift-right: [w263] -> w249
                  shift-left: w248 -> [w264]
                  tunnel: w247 -> [w262] mode=indexing
                  tunnel: [w259] -> w246 mode=indexing
                  n137 = property class="Ring (strict)"(reference=w262, error in=w264) -> (error out=w263:errorcluster, "RingText.Text"=w261:string)  [unwired: 1 out]
                  n138 = Equal?(x="Please Select", y=w261) -> (x = y?=w259:bool)
                }
                n139 = local read "Station Name"() -> (w256:string)
                n140 = Unbundle By Name(w255) -> ("Station Name"=w254:string[])
                n141 = local read "Test Type"() -> (w257:u16)
                n142 = local read "Load?"() -> (w253:bool)
                n143 = Empty String/Path?(string/path=w256) -> (empty?=w244:bool)
                n144 = Search 1D Array(1D array=w254, element=w256) -> (index of element=w252:i32)  [unwired: 1 in]
                n145 = Or Array Elements(Boolean array=w246) -> (logical OR=w245:bool)
                n146 = Select(t=-1, s=w253, f=w252) -> (s? t:f=w251:i32)
                n147 = Or(x=w244, y=w245) -> ()  [unwired: 1 out]
                n148 = case shown="False" w244 {
                  tunnel: [w267 Station_name-state."Idle"] -> w258
                  tunnel: w257 -> [w266 _]
                  tunnel: w251 -> [w265 _]
                  frame False {
                    n149 = case shown="-1" w265 {
                      tunnel: [Station_name-state."Idle" w272] -> w267
                      tunnel: w266 -> [_ w271]
                      frame 0, Default {
                        n150 = One Button Dialog(message="Station name already exist, kindly use other station name.", button name ("OK")="OK") -> ()  [unwired: 1 out]
                      }
                      frame -1 {
                        n151 = case shown="1, Default" w271 {
                          tunnel: [Station_name-state."Idle" w280] -> w272
                          frame 0 {
                            n152 = One Button Dialog(message="Please select Test Type", button name ("OK")="OK") -> ()  [unwired: 1 out]
                          }
                          frame 1, Default {
                            n153 = Two Button Dialog(message="Are you sure to save this setup?", 1:"No" ("F button name (\"Cancel\")"), 2:"Yes" ("T button name (\"OK\")")) -> (T button?=w279:bool)
                            n154 = case shown="True" w279 {
                              tunnel: [Station_name-state."Idle" Station_name-state."Save"] -> w280
                              frame False {
                              }
                              frame True {
                              }
                            }
                          }
                        }
                      }
                    }
                  }
                  frame True {
                    (unwired) "Please insert Station Name" ("message")
                    n155 = One Button Dialog(message="Please insert all field (Station Name and all dropdown in Display section)", button name ("OK")="OK") -> ()  [unwired: 1 out]
                  }
                }
              }
              event "Cancel": Value Change {
                n156 = event-data() -> ()  [unwired: 1 in, 6 out]
                n157 = local write "ForceClose"(TRUE ("ForceClose")) -> ()
              }
              event "Delete": Value Change {
                n158 = event-data() -> ()  [unwired: 1 in, 6 out]
                n159 = Two Button Dialog(message="Are you sure to delete?", 1:"No" ("F button name (\"Cancel\")"), 2:"Yes" ("T button name (\"OK\")")) -> (T button?=→"Delete?":bool)
              }
              event "Test Type": Value Change {
                n160 = event-data() -> ("NewVal"=w297:u16)  [unwired: 1 in]
                n161 = local write "Sub Tab"(w297) -> ()
              }
            }
          }
          frame "Read" {
            n162 = call "Station - Search Serial Number by Device Name.vi"("Ref?"=TRUE, "error in (no error)"=w310, "Array in"=w304) -> ("error out"=w309:errorcluster, "Channel"=w303:i32[], "Index"=w305:i32[])  [unwired: 5 in, 1 out]
            n163 = local read "Sub Tab"() -> (w306:T1)
            n164 = case shown="\"Shearbox\"" w306 {
              tunnel: w305 -> [_ w802 w808 w816 w824 w832 w840 w848 w856 w864 w872]
              tunnel: [w794 w799 w807 w815 w823 w831 w839 w847 w855 w863 w871] -> w308
              tunnel: w303 -> [_ w796 w803 w812 w819 w827 w835 w843 w851 w859 w867]
              tunnel: [w794 w795 w804 w811 w820 w828 w836 w844 w852 w860 w868] -> w302
              frame "Please Select", Default {
                w794 = i32[] []
              }
              frame "Triaxial Shear" {
                n165 = Array Subset(array=w802, index=0, length=6) -> (w799:i32[])
                n166 = Array Subset(array=w796, index=0, length=6) -> (w795:i32[])
              }
              frame "Triaxial UU" {
                n167 = Array Subset(array=w808, index=6, length=4) -> (w807:i32[])
                n168 = Array Subset(array=w803, index=6, length=4) -> (w804:i32[])
              }
              frame "Shearbox" {
                n169 = Array Subset(array=w816, index=10, length=4) -> (w815:i32[])
                n170 = Array Subset(array=w812, index=10, length=4) -> (w811:i32[])
              }
              frame "Permeability" {
                n171 = Array Subset(array=w824, index=14, length=6) -> (w823:i32[])
                n172 = Array Subset(array=w819, index=14, length=6) -> (w820:i32[])
              }
              frame "Consolidation" {
                n173 = Array Subset(array=w832, index=20, length=2) -> (w831:i32[])
                n174 = Array Subset(array=w827, index=20, length=2) -> (w828:i32[])
              }
              frame "Saturation" {
                n175 = Array Subset(array=w840, index=22, length=4) -> (w839:i32[])
                n176 = Array Subset(array=w835, index=22, length=4) -> (w836:i32[])
              }
              frame "User Defined" {
                n177 = Array Subset(array=w848, index=26, length=10) -> (w847:i32[])
                n178 = Array Subset(array=w843, index=26, length=10) -> (w844:i32[])
              }
              frame "UCT" {
                n179 = Array Subset(array=w856, index=36, length=2) -> (w855:i32[])
                n180 = Array Subset(array=w851, index=36, length=2) -> (w852:i32[])
              }
              frame "Iso Consolidation" {
                n181 = Array Subset(array=w864, index=38, length=4) -> (w863:i32[])
                n182 = Array Subset(array=w859, index=38, length=4) -> (w860:i32[])
              }
              frame "Swelling Pressure" {
                n183 = Array Subset(array=w872, index=42, length=2) -> (w871:i32[])
                n184 = Array Subset(array=w867, index=42, length=2) -> (w868:i32[])
              }
            }
            n185 = for {
              shift-right: [w326] -> w307
              shift-left: w309 -> [w322]
              tunnel: w308 -> [w318] mode=indexing
              tunnel: w306 -> [w324]
              tunnel: w302 -> [w313] mode=indexing
              i -> [w325]
              n186 = global read "Global - Channel.vi" "Data"() -> (w321:T10)
              n187 = global read "Global - Unit.vi" "Unit"() -> (w320:T11)
              n188 = Index Array(array=w321, index=w318) -> (element=w323:T12)
              n189 = Index Array(array=w320, index=w318) -> (element=w319:T13)
              n190 = Unbundle By Name(w323) -> ("Channels"=w315:T14)
              n191 = Unbundle By Name(w319) -> ("Unit"=w317:string[], "Decimal Point"=w314:u8[])
              n192 = Cluster To Array(cluster=w315) -> (array=w316:sgl[])
              n193 = case shown="\"Triaxial Shear\"" w324 {
                tunnel: [w327 w334 w395 w438 w481 w542 w567 w610 w653 w750 w775] -> w326
                tunnel: w322 -> [w327 w333 w394 w437 w480 w541 w566 w609 w652 w749 w774]
                tunnel: w325 -> [_ w332 w393 w436 w479 w540 w565 w608 w651 w748 w773]
                tunnel: w316 -> [_ w331 w392 w435 w478 w539 w564 w607 w650 w747 w772]
                tunnel: w317 -> [_ w330 w391 w434 w477 w538 w563 w606 w649 w746 w771]
                tunnel: w314 -> [_ w329 w390 w432 w476 w537 w562 w605 w648 w745 w770]
                tunnel: w313 -> [_ w328 w389 w433 w475 w536 w561 w604 w647 w744 w769]
                frame "Please Select", Default {
                }
                frame "Triaxial Shear" {
                  n194 = case shown="0, Default" w332 {
                    tunnel: [w342 w345 w354 w363 w372 w381] -> w334
                    tunnel: w333 -> [w343 w346 w355 w364 w373 w382]
                    tunnel: w331 -> [w341 w352 w361 w370 w379 w388]
                    tunnel: w330 -> [w340 w351 w360 w369 w378 w387]
                    tunnel: w329 -> [w339 w350 w359 w368 w377 w386]
                    tunnel: w328 -> [w338 w349 w358 w367 w376 w385]
                    frame 0, Default {
                      n195 = Index Array(array=w341, index=w338) -> (element=→"CPT Triaxial Shear":sgl)
                      n196 = Index Array(array=w340, index=w338) -> (element=→"Unit CPT Triaxial Shear":string)
                      n197 = Index Array(array=w339, index=w338) -> (element=w335:u8)
                      n198 = property on="CPT Triaxial Shear" class="DigNum (strict)"(error in=w343, "Precision"=w335) -> (error out=w342:errorcluster)  [unwired: 1 in, 1 out]
                    }
                    frame 1 {
                      n199 = Index Array(array=w352, index=w349) -> (element=→"BPT Triaxial Shear":sgl)
                      n200 = Index Array(array=w351, index=w349) -> (element=→"Unit BPT Triaxial Shear":string)
                      n201 = Index Array(array=w350, index=w349) -> (element=w344:u8)
                      n202 = property on="BPT Triaxial Shear" class="DigNum (strict)"(error in=w346, "Precision"=w344) -> (error out=w345:errorcluster)  [unwired: 1 in, 1 out]
                    }
                    frame 2 {
                      n203 = Index Array(array=w361, index=w358) -> (element=→"VC Triaxial Shear":sgl)
                      n204 = Index Array(array=w360, index=w358) -> (element=→"Unit VC Triaxial Shear":string)
                      n205 = Index Array(array=w359, index=w358) -> (element=w353:u8)
                      n206 = property on="VC Triaxial Shear" class="DigNum (strict)"(error in=w355, "Precision"=w353) -> (error out=w354:errorcluster)  [unwired: 1 in, 1 out]
                    }
                    frame 3 {
                      n207 = Index Array(array=w370, index=w367) -> (element=→"LT Triaxial Shear":sgl)
                      n208 = Index Array(array=w369, index=w367) -> (element=→"Unit LT Triaxial Shear":string)
                      n209 = Index Array(array=w368, index=w367) -> (element=w362:u8)
                      n210 = property on="LT Triaxial Shear" class="DigNum (strict)"(error in=w364, "Precision"=w362) -> (error out=w363:errorcluster)  [unwired: 1 in, 1 out]
                    }
                    frame 4 {
                      n211 = Index Array(array=w379, index=w376) -> (element=→"Disp Triaxial Shear":sgl)
                      n212 = Index Array(array=w378, index=w376) -> (element=→"Unit Disp Triaxial Shear":string)
                      n213 = Index Array(array=w377, index=w376) -> (element=w371:u8)
                      n214 = property on="Disp Triaxial Shear" class="DigNum (strict)"(error in=w373, "Precision"=w371) -> (error out=w372:errorcluster)  [unwired: 1 in, 1 out]
                    }
                    frame 5 {
                      n215 = Index Array(array=w388, index=w385) -> (element=→"PPT Triaxial Shear":sgl)
                      n216 = Index Array(array=w387, index=w385) -> (element=→"Unit PPT Triaxial Shear":string)
                      n217 = Index Array(array=w386, index=w385) -> (element=w380:u8)
                      n218 = property on="PPT Triaxial Shear" class="DigNum (strict)"(error in=w382, "Precision"=w380) -> (error out=w381:errorcluster)  [unwired: 1 in, 1 out]
                    }
                  }
                }
                frame "Triaxial UU" {
                  n219 = case shown="0, Default" w393 {
                    tunnel: [w400 w407 w416 w425] -> w395
                    tunnel: w394 -> [w399 w406 w415 w424]
                    tunnel: w392 -> [w404 w413 w422 w431]
                    tunnel: w391 -> [w403 w412 w421 w430]
                    tunnel: w390 -> [w402 w411 w420 w429]
                    tunnel: w389 -> [w401 w410 w419 w428]
                    frame 0, Default {
                      n220 = Index Array(array=w404, index=w401) -> (element=→"CPT Triaxial UU":sgl)
                      n221 = Index Array(array=w403, index=w401) -> (element=→"Unit CPT Triaxial UU":string)
                      n222 = Index Array(array=w402, index=w401) -> (element=w396:u8)
                      n223 = property on="CPT Triaxial UU" class="DigNum (strict)"(error in=w399, "Precision"=w396) -> (error out=w400:errorcluster)  [unwired: 1 in, 1 out]
                    }
                    frame 1 {
                      n224 = Index Array(array=w413, index=w410) -> (element=→"VLT Triaxial UU":sgl)
                      n225 = Index Array(array=w412, index=w410) -> (element=→"Unit VLT Triaxial UU":string)
                      n226 = Index Array(array=w411, index=w410) -> (element=w405:u8)
                      n227 = property on="VLT Triaxial UU" class="DigNum (strict)"(error in=w406, "Precision"=w405) -> (error out=w407:errorcluster)  [unwired: 1 in, 1 out]
                    }
                    frame 2 {
                      n228 = Index Array(array=w422, index=w419) -> (element=→"Disp Triaxial UU":sgl)
                      n229 = Index Array(array=w421, index=w419) -> (element=→"Unit Disp Triaxial UU":string)
                      n230 = Index Array(array=w420, index=w419) -> (element=w414:u8)
                      n231 = property on="Disp Triaxial UU" class="DigNum (strict)"(error in=w415, "Precision"=w414) -> (error out=w416:errorcluster)  [unwired: 1 in, 1 out]
                    }
                    frame 3 {
                      n232 = Index Array(array=w431, index=w428) -> (element=→"PPT Triaxial UU":sgl)
                      n233 = Index Array(array=w430, index=w428) -> (element=→"Unit PPT Triaxial UU":string)
                      n234 = Index Array(array=w429, index=w428) -> (element=w423:u8)
                      n235 = property on="PPT Triaxial UU" class="DigNum (strict)"(error in=w424, "Precision"=w423) -> (error out=w425:errorcluster)  [unwired: 1 in, 1 out]
                    }
                  }
                }
                frame "Shearbox" {
                  n236 = case shown="3" w436 {
                    tunnel: [w440 w449 w458 w467] -> w438
                    tunnel: w437 -> [w441 w450 w459 w468]
                    tunnel: w435 -> [w447 w456 w465 w474]
                    tunnel: w434 -> [w446 w455 w464 w473]
                    tunnel: w433 -> [w445 w454 w463 w472]
                    tunnel: w432 -> [w444 w453 w462 w471]
                    frame 0, Default {
                      n237 = Index Array(array=w447, index=w445) -> (element=→"LT Shearbox":sgl)
                      n238 = Index Array(array=w446, index=w445) -> (element=→"Unit LT Shearbox":string)
                      n239 = Index Array(array=w444, index=w445) -> (element=w439:u8)
                      n240 = property on="LT Shearbox" class="DigNum (strict)"(error in=w441, "Precision"=w439) -> (error out=w440:errorcluster)  [unwired: 1 in, 1 out]
                    }
                    frame 1 {
                      n241 = Index Array(array=w456, index=w454) -> (element=→"Disp Shearbox":sgl)
                      n242 = Index Array(array=w455, index=w454) -> (element=→"Unit Disp Shearbox":string)
                      n243 = Index Array(array=w453, index=w454) -> (element=w448:u8)
                      n244 = property on="Disp Shearbox" class="DigNum (strict)"(error in=w450, "Precision"=w448) -> (error out=w449:errorcluster)  [unwired: 1 in, 1 out]
                    }
                    frame 2 {
                      n245 = Index Array(array=w465, index=w463) -> (element=→"HLT Shearbox":sgl)
                      n246 = Index Array(array=w464, index=w463) -> (element=→"Unit HLT Shearbox":string)
                      n247 = Index Array(array=w462, index=w463) -> (element=w457:u8)
                      n248 = property on="HLT Shearbox" class="DigNum (strict)"(error in=w459, "Precision"=w457) -> (error out=w458:errorcluster)  [unwired: 1 in, 1 out]
                    }
                    frame 3 {
                      n249 = Index Array(array=w474, index=w472) -> (element=→"H Disp Shearbox":sgl)
                      n250 = Index Array(array=w473, index=w472) -> (element=→"Unit H Dis Shearbox":string)
                      n251 = Index Array(array=w471, index=w472) -> (element=w466:u8)
                      n252 = property on="H Disp Shearbox" class="DigNum (strict)"(error in=w468, "Precision"=w466) -> (error out=w467:errorcluster)  [unwired: 1 in, 1 out]
                    }
                  }
                }
                frame "Permeability" {
                  n253 = case shown="1" w479 {
                    tunnel: [w483 w492 w501 w510 w519 w528] -> w481
                    tunnel: w480 -> [w484 w493 w502 w511 w520 w529]
                    tunnel: w478 -> [w490 w499 w508 w517 w526 w535]
                    tunnel: w477 -> [w489 w498 w507 w516 w525 w534]
                    tunnel: w476 -> [w488 w497 w506 w515 w524 w533]
                    tunnel: w475 -> [w487 w496 w505 w514 w523 w532]
                    frame 0, Default {
                      n254 = Index Array(array=w490, index=w487) -> (element=→"CPT Permeability":sgl)
                      n255 = Index Array(array=w489, index=w487) -> (element=→"Unit CPT Permeability":string)
                      n256 = Index Array(array=w488, index=w487) -> (element=w482:u8)
                      n257 = property on="CPT Permeability" class="DigNum (strict)"(error in=w484, "Precision"=w482) -> (error out=w483:errorcluster)  [unwired: 1 in, 1 out]
                    }
                    frame 1 {
                      n258 = Index Array(array=w499, index=w496) -> (element=→"BPT Permeability":sgl)
                      n259 = Index Array(array=w498, index=w496) -> (element=→"Unit BPT Permeability":string)
                      n260 = Index Array(array=w497, index=w496) -> (element=w491:u8)
                      n261 = property on="BPT Permeability" class="DigNum (strict)"(error in=w493, "Precision"=w491) -> (error out=w492:errorcluster)  [unwired: 1 in, 1 out]
                    }
                    frame 2 {
                      n262 = Index Array(array=w508, index=w505) -> (element=→"IVC Permeability":sgl)
                      n263 = Index Array(array=w507, index=w505) -> (element=→"Unit IVC Permeability":string)
                      n264 = Index Array(array=w506, index=w505) -> (element=w500:u8)
                      n265 = property on="IVC Permeability" class="DigNum (strict)"(error in=w502, "Precision"=w500) -> (error out=w501:errorcluster)  [unwired: 1 in, 1 out]
                    }
                    frame 3 {
                      n266 = Index Array(array=w517, index=w514) -> (element=→"PPT Permeability":sgl)
                      n267 = Index Array(array=w516, index=w514) -> (element=→"Unit PPT Permeability":string)
                      n268 = Index Array(array=w515, index=w514) -> (element=w509:u8)
                      n269 = property on="PPT Permeability" class="DigNum (strict)"(error in=w511, "Precision"=w509) -> (error out=w510:errorcluster)  [unwired: 1 in, 1 out]
                    }
                    frame 4 {
                      n270 = Index Array(array=w526, index=w523) -> (element=→"BPT2 Permeability":sgl)
                      n271 = Index Array(array=w525, index=w523) -> (element=→"Unit BPT2 Permeability":string)
                      n272 = Index Array(array=w524, index=w523) -> (element=w518:u8)
                      n273 = property on="BPT2 Permeability" class="DigNum (strict)"(error in=w520, "Precision"=w518) -> (error out=w519:errorcluster)  [unwired: 1 in, 1 out]
                    }
                    frame 5 {
                      n274 = Index Array(array=w535, index=w532) -> (element=→"OVC Permeability":sgl)
                      n275 = Index Array(array=w534, index=w532) -> (element=→"Unit OVC Permeability":string)
                      n276 = Index Array(array=w533, index=w532) -> (element=w527:u8)
                      n277 = property on="OVC Permeability" class="DigNum (strict)"(error in=w529, "Precision"=w527) -> (error out=w528:errorcluster)  [unwired: 1 in, 1 out]
                    }
                  }
                }
                frame "Consolidation" {
                  n278 = case shown="0, Default" w540 {
                    tunnel: [w544 w554] -> w542
                    tunnel: w541 -> [w545 w553]
                    tunnel: w539 -> [w551 w560]
                    tunnel: w538 -> [w550 w559]
                    tunnel: w537 -> [w549 w558]
                    tunnel: w536 -> [w548 w557]
                    frame 0, Default {
                      n279 = Index Array(array=w551, index=w548) -> (element=→"LT Consolidation":sgl)
                      n280 = Index Array(array=w550, index=w548) -> (element=→"Unit LT Consolidation":string)
                      n281 = Index Array(array=w549, index=w548) -> (element=w543:u8)
                      n282 = property on="LT Consolidation" class="DigNum (strict)"(error in=w545, "Precision"=w543) -> (error out=w544:errorcluster)  [unwired: 1 in, 1 out]
                    }
                    frame 1 {
                      n283 = Index Array(array=w560, index=w557) -> (element=→"Disp Consolidation":sgl)
                      n284 = Index Array(array=w559, index=w557) -> (element=→"Unit Disp Consolidation":string)
                      n285 = Index Array(array=w558, index=w557) -> (element=w552:u8)
                      n286 = property on="Disp Consolidation" class="DigNum (strict)"(error in=w553, "Precision"=w552) -> (error out=w554:errorcluster)  [unwired: 1 in, 1 out]
                    }
                  }
                }
                frame "Saturation" {
                  n287 = case shown="0, Default" w565 {
                    tunnel: [w569 w578 w587 w596] -> w567
                    tunnel: w566 -> [w570 w579 w588 w597]
                    tunnel: w564 -> [w576 w585 w594 w603]
                    tunnel: w563 -> [w575 w584 w593 w602]
                    tunnel: w562 -> [w574 w583 w592 w601]
                    tunnel: w561 -> [w573 w582 w591 w600]
                    frame 0, Default {
                      n288 = Index Array(array=w576, index=w573) -> (element=→"CPT Saturation":sgl)
                      n289 = Index Array(array=w575, index=w573) -> (element=→"Unit CPT Saturation":string)
                      n290 = Index Array(array=w574, index=w573) -> (element=w568:u8)
                      n291 = property on="CPT Saturation" class="DigNum (strict)"(error in=w570, "Precision"=w568) -> (error out=w569:errorcluster)  [unwired: 1 in, 1 out]
                    }
                    frame 1 {
                      n292 = Index Array(array=w585, index=w582) -> (element=→"BPT Saturation":sgl)
                      n293 = Index Array(array=w584, index=w582) -> (element=→"Unit BPT Saturation":string)
                      n294 = Index Array(array=w583, index=w582) -> (element=w577:u8)
                      n295 = property on="BPT Saturation" class="DigNum (strict)"(error in=w579, "Precision"=w577) -> (error out=w578:errorcluster)  [unwired: 1 in, 1 out]
                    }
                    frame 2 {
                      n296 = Index Array(array=w594, index=w591) -> (element=→"VC Saturation":sgl)
                      n297 = Index Array(array=w593, index=w591) -> (element=→"Unit VC Saturation":string)
                      n298 = Index Array(array=w592, index=w591) -> (element=w586:u8)
                      n299 = property on="VC Saturation" class="DigNum (strict)"(error in=w588, "Precision"=w586) -> (error out=w587:errorcluster)  [unwired: 1 in, 1 out]
                    }
                    frame 3 {
                      n300 = Index Array(array=w603, index=w600) -> (element=→"PPT Saturation":sgl)
                      n301 = Index Array(array=w602, index=w600) -> (element=→"Unit PPT Saturation":string)
                      n302 = Index Array(array=w601, index=w600) -> (element=w595:u8)
                      n303 = property on="PPT Saturation" class="DigNum (strict)"(error in=w597, "Precision"=w595) -> (error out=w596:errorcluster)  [unwired: 1 in, 1 out]
                    }
                  }
                }
                frame "Iso Consolidation" {
                  n304 = case shown="3" w608 {
                    tunnel: [w614 w623 w632 w641] -> w610
                    tunnel: w609 -> [w615 w624 w633 w642]
                    tunnel: w607 -> [w619 w628 w637 w646]
                    tunnel: w606 -> [w618 w627 w636 w645]
                    tunnel: w605 -> [w617 w626 w635 w644]
                    tunnel: w604 -> [w616 w625 w634 w643]
                    frame 0, Default {
                      n305 = Index Array(array=w619, index=w616) -> (element=→"CPT iIsoCons":sgl)
                      n306 = Index Array(array=w618, index=w616) -> (element=→"Unit CPT IsoCons":string)
                      n307 = Index Array(array=w617, index=w616) -> (element=w613:u8)
                      n308 = property on="CPT iIsoCons" class="DigNum (strict)"(error in=w615, "Precision"=w613) -> (error out=w614:errorcluster)  [unwired: 1 in, 1 out]
                    }
                    frame 1 {
                      n309 = Index Array(array=w628, index=w625) -> (element=→"BPT iIsoCons":sgl)
                      n310 = Index Array(array=w627, index=w625) -> (element=→"Unit BPT IsoCons":string)
                      n311 = Index Array(array=w626, index=w625) -> (element=w622:u8)
                      n312 = property on="BPT iIsoCons" class="DigNum (strict)"(error in=w624, "Precision"=w622) -> (error out=w623:errorcluster)  [unwired: 1 in, 1 out]
                    }
                    frame 2 {
                      n313 = Index Array(array=w637, index=w634) -> (element=→"VC iIsoCons":sgl)
                      n314 = Index Array(array=w636, index=w634) -> (element=→"Unit VC IsoCons":string)
                      n315 = Index Array(array=w635, index=w634) -> (element=w631:u8)
                      n316 = property on="VC iIsoCons" class="DigNum (strict)"(error in=w633, "Precision"=w631) -> (error out=w632:errorcluster)  [unwired: 1 in, 1 out]
                    }
                    frame 3 {
                      n317 = Index Array(array=w646, index=w643) -> (element=→"PPT iIsoCons":sgl)
                      n318 = Index Array(array=w645, index=w643) -> (element=→"Unit PPT IsoCons":string)
                      n319 = Index Array(array=w644, index=w643) -> (element=w640:u8)
                      n320 = property on="PPT iIsoCons" class="DigNum (strict)"(error in=w642, "Precision"=w640) -> (error out=w641:errorcluster)  [unwired: 1 in, 1 out]
                    }
                  }
                }
                frame "User Defined" {
                  n321 = case shown="4" w651 {
                    tunnel: [w655 w664 w673 w682 w691 w700 w709 w718 w727 w736] -> w653
                    tunnel: w652 -> [w656 w665 w674 w683 w692 w701 w710 w719 w728 w737]
                    tunnel: w650 -> [w662 w671 w680 w689 w698 w707 w716 w725 w734 w743]
                    tunnel: w649 -> [w661 w670 w679 w688 w697 w706 w715 w724 w733 w742]
                    tunnel: w648 -> [w660 w669 w678 w687 w696 w705 w714 w723 w732 w741]
                    tunnel: w647 -> [w659 w668 w677 w686 w695 w704 w713 w722 w731 w740]
                    frame 0, Default {
                      n322 = Index Array(array=w662, index=w659) -> (element=→"CPT User Defined":sgl)
                      n323 = Index Array(array=w661, index=w659) -> (element=→"Unit CPT User Defined":string)
                      n324 = Index Array(array=w660, index=w659) -> (element=w654:u8)
                      n325 = property on="CPT User Defined" class="DigNum (strict)"(error in=w656, "Precision"=w654) -> (error out=w655:errorcluster)  [unwired: 1 in, 1 out]
                    }
                    frame 1 {
                      n326 = Index Array(array=w671, index=w668) -> (element=→"BPT User Defined":sgl)
                      n327 = Index Array(array=w670, index=w668) -> (element=→"Unit BPT User Defined":string)
                      n328 = Index Array(array=w669, index=w668) -> (element=w663:u8)
                      n329 = property on="BPT User Defined" class="DigNum (strict)"(error in=w665, "Precision"=w663) -> (error out=w664:errorcluster)  [unwired: 1 in, 1 out]
                    }
                    frame 2 {
                      n330 = Index Array(array=w680, index=w677) -> (element=→"VC1 User Defined":sgl)
                      n331 = Index Array(array=w679, index=w677) -> (element=→"Unit VC1 User Defined":string)
                      n332 = Index Array(array=w678, index=w677) -> (element=w672:u8)
                      n333 = property on="VC1 User Defined" class="DigNum (strict)"(error in=w674, "Precision"=w672) -> (error out=w673:errorcluster)  [unwired: 1 in, 1 out]
                    }
                    frame 3 {
                      n334 = Index Array(array=w689, index=w686) -> (element=→"PWP User Defined":sgl)
                      n335 = Index Array(array=w688, index=w686) -> (element=→"Unit PWP User Defined":string)
                      n336 = Index Array(array=w687, index=w686) -> (element=w681:u8)
                      n337 = property on="PWP User Defined" class="DigNum (strict)"(error in=w683, "Precision"=w681) -> (error out=w682:errorcluster)  [unwired: 1 in, 1 out]
                    }
                    frame 4 {
                      n338 = Index Array(array=w698, index=w695) -> (element=→"BPT2 User Defined":sgl)
                      n339 = Index Array(array=w697, index=w695) -> (element=→"Unit BPT2 User Defined":string)
                      n340 = Index Array(array=w696, index=w695) -> (element=w690:u8)
                      n341 = property on="BPT2 User Defined" class="DigNum (strict)"(error in=w692, "Precision"=w690) -> (error out=w691:errorcluster)  [unwired: 1 in, 1 out]
                    }
                    frame 5 {
                      n342 = Index Array(array=w707, index=w704) -> (element=→"VC2 User Defined":sgl)
                      n343 = Index Array(array=w706, index=w704) -> (element=→"Unit VC2 User Defined":string)
                      n344 = Index Array(array=w705, index=w704) -> (element=w699:u8)
                      n345 = property on="VC2 User Defined" class="DigNum (strict)"(error in=w701, "Precision"=w699) -> (error out=w700:errorcluster)  [unwired: 1 in, 1 out]
                    }
                    frame 6 {
                      n346 = Index Array(array=w716, index=w713) -> (element=→"VL User Defined":sgl)
                      n347 = Index Array(array=w715, index=w713) -> (element=→"Unit VL User Defined":string)
                      n348 = Index Array(array=w714, index=w713) -> (element=w708:u8)
                      n349 = property on="VL User Defined" class="DigNum (strict)"(error in=w710, "Precision"=w708) -> (error out=w709:errorcluster)  [unwired: 1 in, 1 out]
                    }
                    frame 7 {
                      n350 = Index Array(array=w725, index=w722) -> (element=→"VD User Defined":sgl)
                      n351 = Index Array(array=w724, index=w722) -> (element=→"Unit VD User Defined":string)
                      n352 = Index Array(array=w723, index=w722) -> (element=w717:u8)
                      n353 = property on="VD User Defined" class="DigNum (strict)"(error in=w719, "Precision"=w717) -> (error out=w718:errorcluster)  [unwired: 1 in, 1 out]
                    }
                    frame 8 {
                      n354 = Index Array(array=w734, index=w731) -> (element=→"HL User Defined":sgl)
                      n355 = Index Array(array=w733, index=w731) -> (element=→"Unit HL User Defined":string)
                      n356 = Index Array(array=w732, index=w731) -> (element=w726:u8)
                      n357 = property on="HL User Defined" class="DigNum (strict)"(error in=w728, "Precision"=w726) -> (error out=w727:errorcluster)  [unwired: 1 in, 1 out]
                    }
                    frame 9 {
                      n358 = Index Array(array=w743, index=w740) -> (element=→"HD User Defined":sgl)
                      n359 = Index Array(array=w742, index=w740) -> (element=→"Unit HD User Defined":string)
                      n360 = Index Array(array=w741, index=w740) -> (element=w735:u8)
                      n361 = property on="HD User Defined" class="DigNum (strict)"(error in=w737, "Precision"=w735) -> (error out=w736:errorcluster)  [unwired: 1 in, 1 out]
                    }
                  }
                }
                frame "UCT" {
                  n362 = case shown="1" w748 {
                    tunnel: [w754 w764] -> w750
                    tunnel: w749 -> [w755 w763]
                    tunnel: w747 -> [w759 w768]
                    tunnel: w746 -> [w758 w767]
                    tunnel: w745 -> [w757 w766]
                    tunnel: w744 -> [w756 w765]
                    frame 0, Default {
                      n363 = Index Array(array=w759, index=w756) -> (element=→"LT iUCT":sgl)
                      n364 = Index Array(array=w758, index=w756) -> (element=→"Unit LT UCT":string)
                      n365 = Index Array(array=w757, index=w756) -> (element=w753:u8)
                      n366 = property on="LT iUCT" class="DigNum (strict)"(error in=w755, "Precision"=w753) -> (error out=w754:errorcluster)  [unwired: 1 in, 1 out]
                    }
                    frame 1 {
                      n367 = Index Array(array=w768, index=w765) -> (element=→"Disp iUCT":sgl)
                      n368 = Index Array(array=w767, index=w765) -> (element=→"Unit Disp UCT":string)
                      n369 = Index Array(array=w766, index=w765) -> (element=w762:u8)
                      n370 = property on="Disp iUCT" class="DigNum (strict)"(error in=w763, "Precision"=w762) -> (error out=w764:errorcluster)  [unwired: 1 in, 1 out]
                    }
                  }
                }
                frame "Swelling Pressure" {
                  n371 = case shown="0, Default" w773 {
                    tunnel: [w779 w789] -> w775
                    tunnel: w774 -> [w780 w788]
                    tunnel: w772 -> [w784 w793]
                    tunnel: w771 -> [w783 w792]
                    tunnel: w770 -> [w782 w791]
                    tunnel: w769 -> [w781 w790]
                    frame 0, Default {
                      n372 = Index Array(array=w784, index=w781) -> (element=→"VL SP":sgl)
                      n373 = Index Array(array=w783, index=w781) -> (element=→"Unit VL SP":string)
                      n374 = Index Array(array=w782, index=w781) -> (element=w778:u8)
                      n375 = property on="VL SP" class="DigNum (strict)"(error in=w780, "Precision"=w778) -> (error out=w779:errorcluster)  [unwired: 1 in, 1 out]
                    }
                    frame 1 {
                      n376 = Index Array(array=w793, index=w790) -> (element=→"VS SP":sgl)
                      n377 = Index Array(array=w792, index=w790) -> (element=→"Unit VS SP":string)
                      n378 = Index Array(array=w791, index=w790) -> (element=w787:u8)
                      n379 = property on="VS SP" class="DigNum (strict)"(error in=w788, "Precision"=w787) -> (error out=w789:errorcluster)  [unwired: 1 in, 1 out]
                    }
                  }
                }
              }
            }
          }
          frame "Save" {
            n380 = for {
              shift-right: [w909] -> w879
              shift-left: w896 -> [w910]
              tunnel: w895 -> [w908] mode=indexing
              tunnel: [w907] -> w894 mode=indexing
              n381 = property class="Ring (strict)"(reference=w908, error in=w910) -> (error out=w909:errorcluster, "RingText.Text"=w907:string)  [unwired: 1 out]
            }
            n382 = Unbundle By Name(w886) -> ("Station ID"=w885:i32)
            n383 = Number To Decimal String(number=w885) -> (decimal integer string=w884:string)  [unwired: 1 in]
            n384 = for {
              shift-right: [w905] -> w878
              shift-left: w879 -> [w906]
              tunnel: w877 -> [w904] mode=indexing
              tunnel: [w903] -> w876 mode=indexing
              n385 = property class="Ring (strict)"(reference=w904, error in=w906) -> (error out=w905:errorcluster, "RingText.Text"=w903:string)  [unwired: 1 out]
            }
            n386 = local read "Sub Tab"() -> (w887:T1)
            n387 = case shown="\"Swelling Pressure\"" w887 {
              tunnel: [string[] [] w919 w932 w945 w958 w971 w984 w997 w1010 w1023 w1034] -> w883
              tunnel: w894 -> [_ w925 w936 w949 w962 w975 w988 w1001 w1014 w1027 _]
              tunnel: [string[] [] w913 w926 w939 w954 w965 w978 w991 w1004 w1017 w1030] -> w893
              tunnel: w876 -> [_ w916 w929 w942 w953 w968 w981 w994 w1007 w1020 w1031]
              frame "Please Select", Default {
              }
              frame "Triaxial Shear" {
                n388 = Array Subset(array=w925, index=0, length=3) -> (w914:string[])
                n389 = Array Subset(array=w916, index=0, length=6) -> (w915:string[])
                n390 = Build Array (concatenate)(string[] ["Test Type", "CPC Triaxial Shear", "BPC Triaxial Shear", "VLC Triaxial Shear"], string[] ["CP TS", "BP TS", "VL TS", "LT TS", "Disp TS", "PP TS"], "Status" ("String")) -> (w919:string[])
                n391 = Build Array (concatenate)(w914, w915) -> (w913:string[])
              }
              frame "Triaxial UU" {
                n392 = Array Subset(array=w936, index=3, length=2) -> (w927:string[])
                n393 = Array Subset(array=w929, index=6, length=4) -> (w928:string[])
                n394 = Build Array (concatenate)(w927, w928) -> (w926:string[])
                n395 = Build Array (concatenate)(string[] ["Test Type", "CPC Triaxial UU", "VLC Triaxial UU"], string[] ["CP TUU", "VL TUU", "Disp TUU", "PP TUU"], "Status" ("String")) -> (w932:string[])
              }
              frame "Shearbox" {
                n396 = Array Subset(array=w949, index=5, length=2) -> (w940:string[])
                n397 = Array Subset(array=w942, index=10, length=4) -> (w941:string[])
                n398 = Build Array (concatenate)(string[] ["Test Type", "VLC Shearbox", "HLC Shearbox"], string[] ["VL Shearbox", "VDisp Shearbox", "HL Shearbox", "HDisp Shearbox"], "Status" ("String")) -> (w945:string[])
                n399 = Build Array (concatenate)(w940, w941) -> (w939:string[])
              }
              frame "Permeability" {
                n400 = Array Subset(array=w962, index=7, length=3) -> (w955:string[])
                n401 = Array Subset(array=w953, index=14, length=6) -> (w952:string[])
                n402 = Build Array (concatenate)(string[] ["Test Type", "CPC Permeability", "BPC Permeability", "BPC2 Permeability"], string[] ["CP Permea", "BP Permea", "IVC Permea", "PP Permea", "BP2 Permea", "OVC Permea"], "Status" ("String")) -> (w958:string[])
                n403 = Build Array (concatenate)(w955, w952) -> (w954:string[])
              }
              frame "Consolidation" {
                n404 = Array Subset(array=w975, index=10, length=1) -> (w966:string[])
                n405 = Array Subset(array=w968, index=20, length=2) -> (w967:string[])
                n406 = Build Array (concatenate)(w966, w967) -> (w965:string[])
                n407 = Build Array (concatenate)(string[] ["Test Type", "VLC Consolidation"], string[] ["LT Consol", "Disp Consol"], "Status" ("String")) -> (w971:string[])
              }
              frame "Saturation" {
                n408 = Array Subset(array=w988, index=11, length=2) -> (w979:string[])
                n409 = Array Subset(array=w981, index=22, length=4) -> (w980:string[])
                n410 = Build Array (concatenate)(string[] ["Test Type", "CPC Saturation", "BPC Saturation"], string[] ["CP Saturation", "BP Saturation", "VC Saturation", "PP Saturation"], "Status" ("String")) -> (w984:string[])
                n411 = Build Array (concatenate)(w979, w980) -> (w978:string[])
              }
              frame "User Defined" {
                n412 = Array Subset(array=w1001, index=13, length=5) -> (w992:string[])
                n413 = Array Subset(array=w994, index=26, length=10) -> (w993:string[])
                n414 = Build Array (concatenate)(string[] ["Test Type", "CPC User Defined", "BPC User Defined", "BPC2 User Defined", "VLC User Defined", "HLC User Defined"], string[] ["CP UD", "BP UD", "VC1 UD", "PP UD", "BP2 UD", "VC2 UD", "VL UD", "VDisp UD", "HL UD", "H Disp UD"], "Status" ("String")) -> (w997:string[])
                n415 = Build Array (concatenate)(w992, w993) -> (w991:string[])
              }
              frame "UCT" {
                n416 = Array Subset(array=w1014, index=18, length=1) -> (w1005:string[])
                n417 = Array Subset(array=w1007, index=36, length=2) -> (w1006:string[])
                n418 = Build Array (concatenate)(w1005, w1006) -> (w1004:string[])
                n419 = Build Array (concatenate)(string[] ["Test Type", "VLC UCT"], string[] ["LT UCT", "Disp UCT"], "Status" ("String")) -> (w1010:string[])
              }
              frame "Iso Consolidation" {
                n420 = Array Subset(array=w1027, index=19, length=2) -> (w1018:string[])
                n421 = Array Subset(array=w1020, index=38, length=4) -> (w1019:string[])
                n422 = Build Array (concatenate)(string[] ["Test Type", "CPC Iso", "BPC Iso"], string[] ["CP Iso", "BP Iso", "VC Iso", "PP Iso"], "Status" ("String")) -> (w1023:string[])
                n423 = Build Array (concatenate)(w1018, w1019) -> (w1017:string[])
              }
              frame "Swelling Pressure" {
                n424 = Array Subset(array=w1031, index=42, length=2) -> (w1030:string[])
                n425 = Build Array (concatenate)(string[] ["Test Type"], string[] ["VL SPres", "VS SPres"], "Status" ("String")) -> (w1034:string[])
              }
            }
            n426 = property on="Test Type" class="Ring (strict)"(error in=w878) -> (error out=w898:errorcluster, "RingText.Text"=w892:string)  [unwired: 1 in, 1 out]
            n427 = Insert Into Array(array=w893, index=0, new element #1=w892, new element #2=w884) -> (w889:string[])
            n428 = local read "Station Name"() -> (w875:string)
            n429 = Insert Into Array(array=w883, index=1, new element="ID" ("new element/subarray")) -> (w882:string[])
            n430 = Build Array (concatenate)(w889, "0" ("String")) -> (w888:string[])
            n431 = To Upper Case(1:w875) -> (0:w897:string)
            n432 = call "Station - Config File.vi"("Action"=enum16{"Write", "Read", "Read All", "Remove"}."Write", "error in (no error)"=w898, "Value"=w888, "Key Name"=w882, "Station Name"=w897) -> ("error out"=w899:errorcluster)  [unwired: 5 in, 1 out]
            n433 = case shown="No Error" w899 {
              selector: w899 -> [w1039 _]
              tunnel: [w1039 errorcluster {"status"=FALSE, "code"=0, "source"=""} ("error IO")] -> w902
              tunnel: [Station_name-state."Close" Station_name-state."Idle"] -> w901
              frame No Error {
                n434 = One Button Dialog(message="Save succesful..") -> ()  [unwired: 1 in, 1 out]
              }
              frame Error {
                n435 = One Button Dialog(message="Save not success..") -> ()  [unwired: 1 in, 1 out]
              }
            }
          }
          frame "Load" {
            n436 = local read "Sub Tab"() -> (w1051:T1)
            n437 = case shown="\"Iso Consolidation\"" w1051 {
              tunnel: [string[] [] w1080 w1093 w1106 w1119 w1132 w1145 w1158 w1171 w1184] -> w1048
              tunnel: w1050 -> [_ w1086 w1097 w1110 w1123 w1136 w1149 w1162 w1175 w1188]
              tunnel: [refnum<vi>[] [] w1074 w1087 w1100 w1115 w1126 w1139 w1152 w1165 w1178] -> w1047
              tunnel: w1049 -> [_ w1077 w1090 w1103 w1114 w1129 w1142 w1155 w1168 w1181]
              frame "Please Select", Default {
              }
              frame "Triaxial Shear" {
                n438 = Array Subset(array=w1086, index=0, length=3) -> (w1075:refnum<vi>[])
                n439 = Array Subset(array=w1077, index=0, length=6) -> (w1076:refnum<vi>[])
                n440 = Build Array (concatenate)(string[] ["Test Type", "CPC Triaxial Shear", "BPC Triaxial Shear", "VLC Triaxial Shear"], string[] ["CPC TS", "BPC TS", "VLC TS", "LT TS", "Disp TS", "PP TS"], "Status" ("String")) -> (w1080:string[])
                n441 = Build Array (concatenate)(w1075, w1076) -> (w1074:refnum<vi>[])
              }
              frame "Triaxial UU" {
                n442 = Array Subset(array=w1097, index=3, length=2) -> (w1088:refnum<vi>[])
                n443 = Array Subset(array=w1090, index=6, length=4) -> (w1089:refnum<vi>[])
                n444 = Build Array (concatenate)(w1088, w1089) -> (w1087:refnum<vi>[])
                n445 = Build Array (concatenate)(string[] ["Test Type", "CPC Triaxial UU", "VLC Triaxial UU"], string[] ["CPC TUU", "VLC TUU", "Disp TUU", "PP TUU"], "Status" ("String")) -> (w1093:string[])
              }
              frame "Shearbox" {
                n446 = Array Subset(array=w1110, index=5, length=2) -> (w1101:refnum<vi>[])
                n447 = Array Subset(array=w1103, index=10, length=4) -> (w1102:refnum<vi>[])
                n448 = Build Array (concatenate)(string[] ["Test Type", "VLC Shearbox", "HLC Shearbox"], string[] ["VL Shearbox", "VDisp Shearbox", "HL Shearbox", "HDisp Shearbox"], "Status" ("String")) -> (w1106:string[])
                n449 = Build Array (concatenate)(w1101, w1102) -> (w1100:refnum<vi>[])
              }
              frame "Permeability" {
                n450 = Array Subset(array=w1123, index=7, length=3) -> (w1116:refnum<vi>[])
                n451 = Array Subset(array=w1114, index=14, length=6) -> (w1113:refnum<vi>[])
                n452 = Build Array (concatenate)(string[] ["Test Type", "CPC Permeability", "BPC Permeability", "BPC2 Permeability"], string[] ["CP Permea", "BP Permea", "IVC Permea", "PP Permea", "BP2 Permea", "OVC Permea"], "Status" ("String")) -> (w1119:string[])
                n453 = Build Array (concatenate)(w1116, w1113) -> (w1115:refnum<vi>[])
              }
              frame "Consolidation" {
                n454 = Array Subset(array=w1136, index=10, length=1) -> (w1127:refnum<vi>[])
                n455 = Array Subset(array=w1129, index=20, length=2) -> (w1128:refnum<vi>[])
                n456 = Build Array (concatenate)(w1127, w1128) -> (w1126:refnum<vi>[])
                n457 = Build Array (concatenate)(string[] ["Test Type", "VLC Consolidation"], string[] ["LT Consol", "Disp Consol"], "Status" ("String")) -> (w1132:string[])
              }
              frame "Saturation" {
                n458 = Array Subset(array=w1149, index=11, length=2) -> (w1140:refnum<vi>[])
                n459 = Array Subset(array=w1142, index=22, length=4) -> (w1141:refnum<vi>[])
                n460 = Build Array (concatenate)(string[] ["Test Type", "CPC Saturation", "BPC Saturation"], string[] ["CP Saturation", "BP Saturation", "VC Saturation", "PP Saturation"], "Status" ("String")) -> (w1145:string[])
                n461 = Build Array (concatenate)(w1140, w1141) -> (w1139:refnum<vi>[])
              }
              frame "User Defined" {
                n462 = Array Subset(array=w1162, index=13, length=5) -> (w1153:refnum<vi>[])
                n463 = Array Subset(array=w1155, index=26, length=10) -> (w1154:refnum<vi>[])
                n464 = Build Array (concatenate)(string[] ["Test Type", "CPC User Defined", "BPC User Defined", "BPC2 User Defined", "VLC User Defined", "HLC User Defined"], string[] ["CP UD", "BP UD", "VC1 UD", "PP UD", "BP2 UD", "VC2 UD", "VL UD", "VDisp UD", "HL UD", "H Disp UD"], "Status" ("String")) -> (w1158:string[])
                n465 = Build Array (concatenate)(w1153, w1154) -> (w1152:refnum<vi>[])
              }
              frame "UCT" {
                n466 = Array Subset(array=w1175, index=18, length=1) -> (w1166:refnum<vi>[])
                n467 = Array Subset(array=w1168, index=36, length=2) -> (w1167:refnum<vi>[])
                n468 = Build Array (concatenate)(w1166, w1167) -> (w1165:refnum<vi>[])
                n469 = Build Array (concatenate)(string[] ["Test Type", "VLC Consolidation"], string[] ["LT Consol", "Disp Consol"], "Status" ("String")) -> (w1171:string[])
              }
              frame "Iso Consolidation" {
                n470 = Array Subset(array=w1188, index=19, length=2) -> (w1179:refnum<vi>[])
                n471 = Array Subset(array=w1181, index=38, length=4) -> (w1180:refnum<vi>[])
                n472 = Build Array (concatenate)(string[] ["Test Type", "CPC Saturation", "BPC Saturation"], string[] ["CP Saturation", "BP Saturation", "VC Saturation", "PP Saturation"], "Status" ("String")) -> (w1184:string[])
                n473 = Build Array (concatenate)(w1179, w1180) -> (w1178:refnum<vi>[])
              }
            }
            n474 = local read "Station Name"() -> (w1054:string)
            n475 = call "Station - Config File.vi"("Action"=enum16{"Write", "Read", "Read All", "Remove"}."Read", "error in (no error)"=w1055, "Key Name"=w1048, "Station Name"=w1054) -> ("error out"=w1059:errorcluster, "Value Out"=w1066:T7)  [unwired: 6 in]
            n476 = Index Array(array=w1066) -> (element=w1065:T15)  [unwired: 1 in]
            n477 = Unbundle By Name(w1065) -> ("Key Value"=w1064:string[])
            n478 = Delete From Array(array=w1064) -> (array with subset deleted=w1063:string[])  [unwired: 2 in, 1 out]
            n479 = Delete From Array(array=w1063, length=2, index=0) -> (deleted portion=w1058:string[], array with subset deleted=w1060:string[])
            "List" <- w1060
            n480 = Index Array(array=w1058, index=1) -> (element=→"Station ID":string)
            n481 = global read "Global - Device.vi" "Device"() -> (w1045:string[])
            n482 = for {
              tunnel: w1045 -> [w1071] mode=indexing
              tunnel: [w1071] -> w1044 mode=indexing if=w1069
              n483 = Empty String/Path?(string/path=w1071) -> (empty?=w1070:bool)
              n484 = Not(x=w1070) -> (.not. x?=w1069:bool)
            }
            "Device" <- w1044
            n485 = global read "Global - Device Input.vi" "Device Input"() -> (w1046:string[])
            n486 = for {
              tunnel: w1060 -> [w1191] mode=indexing
              tunnel: w1044 -> [w1194]
              shift-right: [w1201] -> w1052
              shift-left: w1059 -> [w1202]
              tunnel: w1047 -> [w1200] mode=indexing
              tunnel: w1046 -> [w1193]
              n487 = Match Pattern(string=w1191, regular expression=" | ") -> (after substring=w1196:string)  [unwired: 1 in, 3 out]
              n488 = Empty String/Path?(string/path=w1196) -> (empty?=w1195:bool)
              n489 = Select(t=w1194, s=w1195, f=w1193) -> (s? t:f=w1192:string[])
              n490 = Search 1D Array(1D array=w1192, element=w1191) -> (index of element=w1199:i32)  [unwired: 1 in]
              n491 = Increment(x=w1199) -> (x+1=w1198:i32)
              n492 = property class="Ring (strict)"(reference=w1200, error in=w1202, "Value"=w1198) -> (error out=w1201:errorcluster)  [unwired: 1 out]
            }
          }
          frame "Close" {
          }
        }
      }
      frame Error {
      }
    }
  }
  "error out" <- w37
